vi "Phase III control screen - modified EPV.vi"() -> ()   [LabVIEW 2020]
uses:
  UI Message handler/User Event - Stop/User Event - Stop.lvlib
  UI Message handler/Message Queue/Message Queue.lvlib
  Globals/Phase III Globals.vi
  Controls/boolean ref.ctl
  Controls/Config.ctl
  Controls/EPV .ctl
panel:
  out "Login screen cover":bool
  in  "Log In Tool":bool
  out "User 3":string
  out "User 2":string
  out "State LOX":dbl(knob) caption="Gauge" scale=0.0..40000.0
  out "State ATF":dbl(knob) caption="Gauge" scale=0.0..40000.0
  out "User":string
  in  "C_EPV_124":bool
  out "C_EPV_124 HSS":bool
  in  "C_EPV_16":bool
  in  "N_EPV_202":bool
  in  "C_EPV_1352":bool
  in  "C_EPV_18":bool
  in  "C_EPV_803":bool
  in  "N_EPV_141":bool
  in  "G_EPV_51":bool
  in  "N_EPV_61":bool
  in  "N_EPV_62b":bool
  in  "N_EPV_62a":bool
  in  "C_EPV_127":bool
  in  "C_EPV_123":bool
  in  "C_EPV_8":bool
  in  "C_EPV_7":bool
  in  "C_EPV_2":bool
  in  "F_EPV_75":bool
  in  "N_EPV_206":bool
  in  "N_EPV_203":bool
  in  "F_EPV_28":bool
  in  "F_EPV_142":bool
  in  "F_EPV_ 33":bool
  in  "N_EPV_ 69":bool
  in  "N_EPV_68":bool
  in  "F_EPV_41":bool
  in  "F_EPV_21":bool
  in  "F_EPV_132":bool
  in  "F_EPV_136":bool
  in  "F_EPV_131":bool
  in  "Exit RT":bool
  out "PPSU":bool
  out "RUN ACKNOWLEDGE LOX":bool
  out "Shaft Rotational Direction":string
  out "Speed RPM -lox":dbl format="%#_g r/min"
  out "Frequency":dbl format="%#_g Hz"
  in  "SPEED                      l":dbl format="%#_g r/m"
  in  "RAMP DOWN      l":dbl format="%#_g S"
  in  "RAMP UP             l":dbl format="%#_g S"
  in  "SET FREQ             l":dbl format="%#_g Hz"
  out "RUN ACKNOWLEDGE Atf":bool
  out "Shaft Rotational Direction":string
  out "Speed RPM":dbl format="%#_g r/min"
  out "Frequency":dbl format="%#_g Hz"
  out "Terminal Power":dbl format="%#_g W"
  out "Terminal Current":dbl format="%#_g A"
  out "Terminal Voltage":dbl format="%#_g V"
  out "C_EPV_16 HSS":bool
  out "N_EPV_202 HSS":bool
  out "C_EPV_1352 HSS":bool
  out "C_EPV_18 HSS":bool
  out "C_EPV_803 HSS":bool
  out "N_EPV_141 HSS":bool
  out "G_EPV_51 HSS":bool
  out "N_EPV_61 HSS":bool
  out "N_EPV_62b HSS":bool
  out "N_EPV_62a HSS":bool
  out "C_EPV_127 HSS":bool
  out "C_EPV_123 HSS":bool
  out "C_EPV_8 HSS":bool
  out "C_EPV_7 HSS":bool
  out "C_EPV_2 HSS":bool
  out "N_EPV_75 HSS":bool
  out "N_EPV_206 HSS":bool
  out "N_EPV_203 HSS":bool
  out "F_EPV_28 HSS":bool
  out "N_EPV_142 HSS":bool
  out "F_EPV_33 HSS":bool
  out "N_EPV_69 HSS":bool
  out "N_EPV_68 HSS":bool
  out "F_EPV_41 HSS":bool
  out "F_EPV_21 HSS":bool
  out "F_EPV_132 HSS":bool
  out "F_EPV_136 HSS":bool
  out "F_EPV_131 HSS":bool
  out "MS failure":bool
  out "Over power detection":bool
  out "Over current detection":bool
  out "over voltage detection":bool
  out "power failure status":bool
  out "LOG":bool
  out "TARGET":bool
  out "DR L":bool
  out "DR A":bool
  out "DO":bool
  out "DI":bool
  out "AO":bool
  out "AI":bool
  in  "ADC reset ATF":bool
  in  "MCU reset ATF":bool
  in  "Gate driver ATF":bool
  in  "Motor off ATF":bool
  in  "Motor On ATF":bool
  in  "Update drive ATF":bool
  in  "Adc reset lox":bool
  in  "MCU Reset -LOX":bool
  in  "Gate driver- LOX":bool
  in  "DC off":bool
  in  "DC on":bool
  in  "update ppsu":bool
  in  "Motor Off lox":bool
  in  "Motor On lox":bool
  in  "Update drive lox":bool
  in  "STOP LOG":bool
  in  "SPEED":dbl format="%#_g r/m"
  in  "RAMP DOWN":dbl format="%#_g S"
  in  "RAMP UP":dbl format="%#_g S"
  in  "SET FREQ":dbl format="%#_g Hz"
  in  "SET POWER":dbl format="%#_g W"
  in  "SET CURRENT":dbl format="%#_g A"
  in  "SET VOLTAGE":dbl format="%#_g V"
  in  "OPP(W)":dbl format="%#_g W"
  in  "OCP(A)":dbl format="%#_g A"
  in  "OVP(V)":dbl format="%#_g V"
  in  "Ms initialize":bool
  in  "Alarm ack":bool
  in  "Connect Drive Lox":bool
  in  "Connect Drive ATF":bool
  out "Time Stamp":timestamp format="%<%.3X>T"
  in  "Configure IP":bool
  in  "Datalog phase code":string(combo)
  in  "ABORT":bool
  in  "CONFIGURATION FILE":string(combo)
  in  "IP ADDRESS":string
  in  "HOLD UPDATE":bool
  in  "DAQ SETTING":bool
  in  "Connect ppsu":bool
  in  "Connect RT":bool
  in  "STOP DAQ":bool
  in  "EXIT":bool
  in  "START LOG":bool
  in  "START DAQ":bool
  # "VERSION NUMBER : 1.5"
  # "PHASE III"
  # "RELEASE DATE :10/06/2024"
  # "Select the configuration file"
  # "Select the phase code"
  # "+"
  # "SEQUENCE"
  # "ATF"
  # "LOX"
  # "ENGINE"
  # "EPV CONTROLS"
  # "EPV CONTROLS"
  # "EPV CONTROLS"
  # "Drive ATF Controls"
  # "Drive LOX Controls"
  # "PPSU"
  # "DRIVE ATF"
  # "DRIVE LOX"
  # "PPSU Controls"
  # "PPSU FEEDBACK PARAMETER"
  # "DRIVE ATF SET PARAMETER"
  # "Motor Rotational State"
  # "PPSU SET PARAMETER"
  # "DRIVE LOX SET PARAMETER"
  # "Motor Rotational State"
  # "PPSU FEEDBACK PARAMETER"
  # "DRIVE ATF FEEDBACK PARAMETER"
  # "DRIVE ATF FEEDBACK PARAMETER"
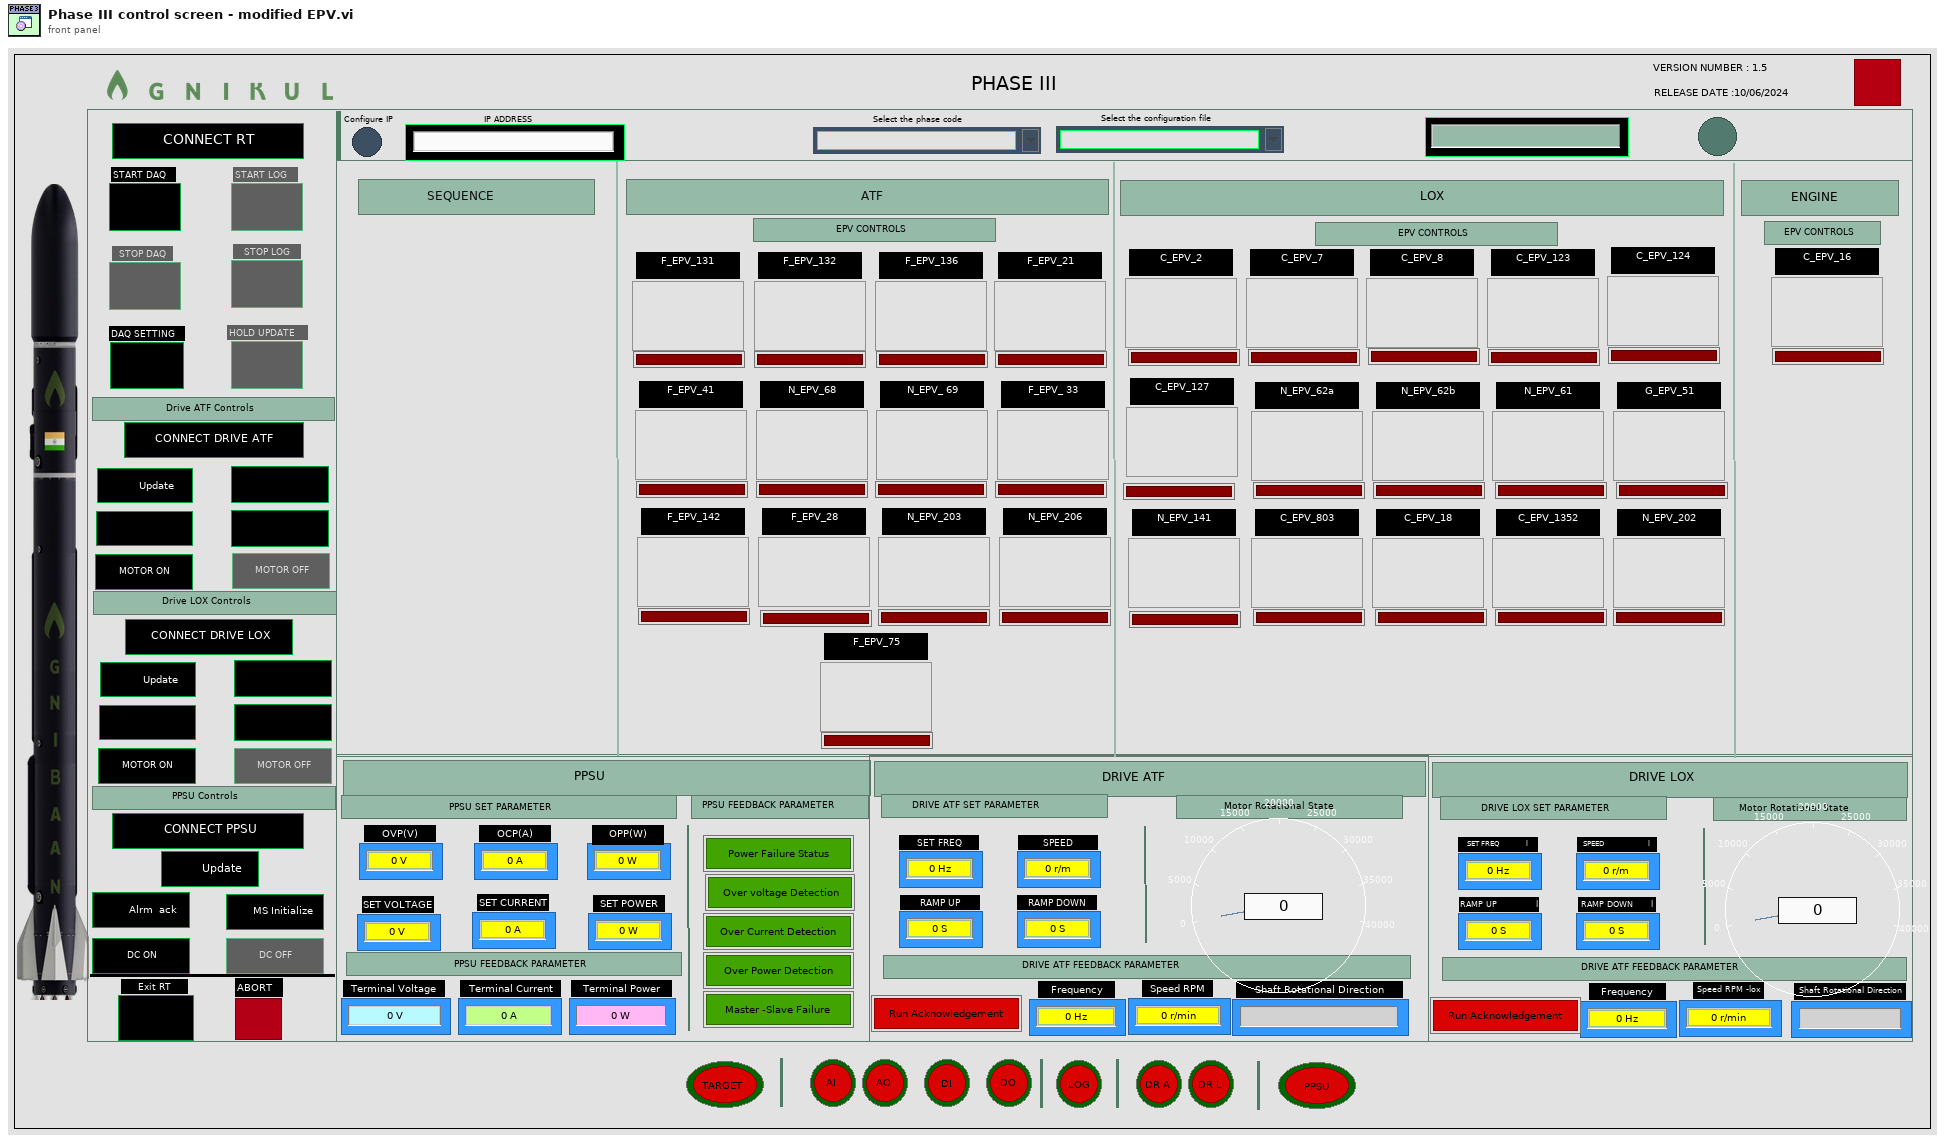
[diagram p1: front panel]
types:
  T1 = typedef "boolean ref.ctl" = cluster{"Connect RT":refnum<vi>, "START DAQ":refnum<vi>, "STOP DAQ":refnum<vi>, "DAQ SETTING":refnum<vi>, "START LOG":refnum<vi>, "STOP LOG":refnum<vi>, "Connect Drive ATF":refnum<vi>, "Update drive ATF":refnum<vi>, "Gate driver ATF":refnum<vi>, "Motor On ATF":refnum<vi>, "ADC reset ATF":refnum<vi>, "Gate driver ATF 2":refnum<vi>, "Motor off ATF":refnum<vi>, "MCU reset ATF":refnum<vi>, "Connect Drive Lox":refnum<vi>, "Update drive lox":refnum<vi>, "Gate driver- LOX":refnum<vi>, "Motor On lox":refnum<vi>, "Adc reset lox":refnum<vi>, "MCU Reset -LOX":refnum<vi>, "Motor Off lox":refnum<vi>, "Connect ppsu":refnum<vi>, "update ppsu":refnum<vi>, "DC on":refnum<vi>, "Alarm ack":refnum<vi>, "DC off":refnum<vi>, "Ms initialize":refnum<vi>, "Exit RT":refnum<vi>, "ABORT":refnum<vi>, "HOLD UPDATE":refnum<vi>}
  T2 = typedef "EPV .ctl" = cluster{"F_EPV_131":refnum<vi>, "F_EPV_132":refnum<vi>, "F_EPV_136":refnum<vi>, "F_EPV_21":refnum<vi>, "F_EPV_41":refnum<vi>, "N_EPV_68":refnum<vi>, "N_EPV_ 69":refnum<vi>, "N_EPV_ 33":refnum<vi>, "F_EPV_142":refnum<vi>, "F_EPV_28":refnum<vi>, "N_EPV_203":refnum<vi>, "N_EPV_206":refnum<vi>, "F_EPV_75":refnum<vi>, "C_EPV_2":refnum<vi>, "C_EPV_7":refnum<vi>, "C_EPV_8":refnum<vi>, "C_EPV_123":refnum<vi>, "C_EPV_124":refnum<vi>, "C_EPV_127":refnum<vi>, "N_EPV_62a":refnum<vi>, "N_EPV_62b":refnum<vi>, "N_EPV_61":refnum<vi>, "G_EPV_51":refnum<vi>, "N_EPV_141":refnum<vi>, "C_EPV_803":refnum<vi>, "C_EPV_18":refnum<vi>, "C_EPV_1352":refnum<vi>, "N_EPV_202":refnum<vi>, "C_EPV_16":refnum<vi>}
  T3 = enum8{"Enabled", "Disabled", "Disabled and Grayed Out"}[]
  T4 = typedef "file folder ctl.ctl" = cluster{"Datalog path":path, "Configuration path":path, "Signal list path":path, "Sub vi's":path, "Authentication":path}
  T5 = typedef "Notifier ctl.ctl" = cluster{"Data":refnum<notifier>}
  T6 = typedef "Message Queue.lvlib/All Message Queues.ctl" = cluster{"UI":refnum<queue>, "NS ":refnum<queue>}
  T7 = typedef "Config.ctl" = cluster{"AO config":cluster{"Channel_Name":string, "Channel_Number":string, "Default_Value":dbl, "Units":string}[], "AI config":cluster{"Channel_Name":string, "Channel_Number":string, "Pre_Scale_min":dbl, "Pre_Scale_max":dbl, "Sensor_min":dbl, "Sensor_max":dbl, "Units":string}[], "DI config":cluster{"Channel_Name":string, "Channel_Number":string, "Default_Value":bool, "DI invert?":bool}[], "DO config":cluster{"Channel_Name":string, "Channel_Number":string, "Default_Value":bool, "DO invert?":bool}[], "TC config":cluster{"Channel_Name":string, "Channel_Number":string, "Pre_Scale_min":dbl, "Pre_Scale_max":dbl, "units":i32, " type":i32}[], "ACC config":cluster{"Channel_Name":string, "Channel_Number":string, "Pre_Scale_min":dbl, "Pre_Scale_max":dbl, "Terminal configuration":i32, "Sensitivity":dbl, "Sensitivity units":i32}[], "SG config":cluster{"Channel_Name":string, "Channel_Number":string, "Pre_Scale_min":dbl, "Pre_Scale_max":dbl}[], "Strain Gauge Settings":cluster{"poisson ratio":dbl, "nominal gage resistance":dbl, "gage factor":dbl}, "Bridge Settings":cluster{"voltage excitation value":dbl, "voltage excitation source":i32, "initial bridge voltage":dbl, "lead wire resistance":dbl, "strain configuration":i32}, "Sample Rate":cluster{"AI Sample Rate":dbl[], "AO Sample Rate":dbl[], "DI Sample Rate":dbl[], "TC Sample Rate":dbl[], "DO Sample Rate":dbl[], "SG Sample Rate":dbl[], "ACC Sample Rate":dbl[]}}
  T8 = enum16{"open", "replace", "create", "open or create", "replace or create", "replace or create with confirmation"}
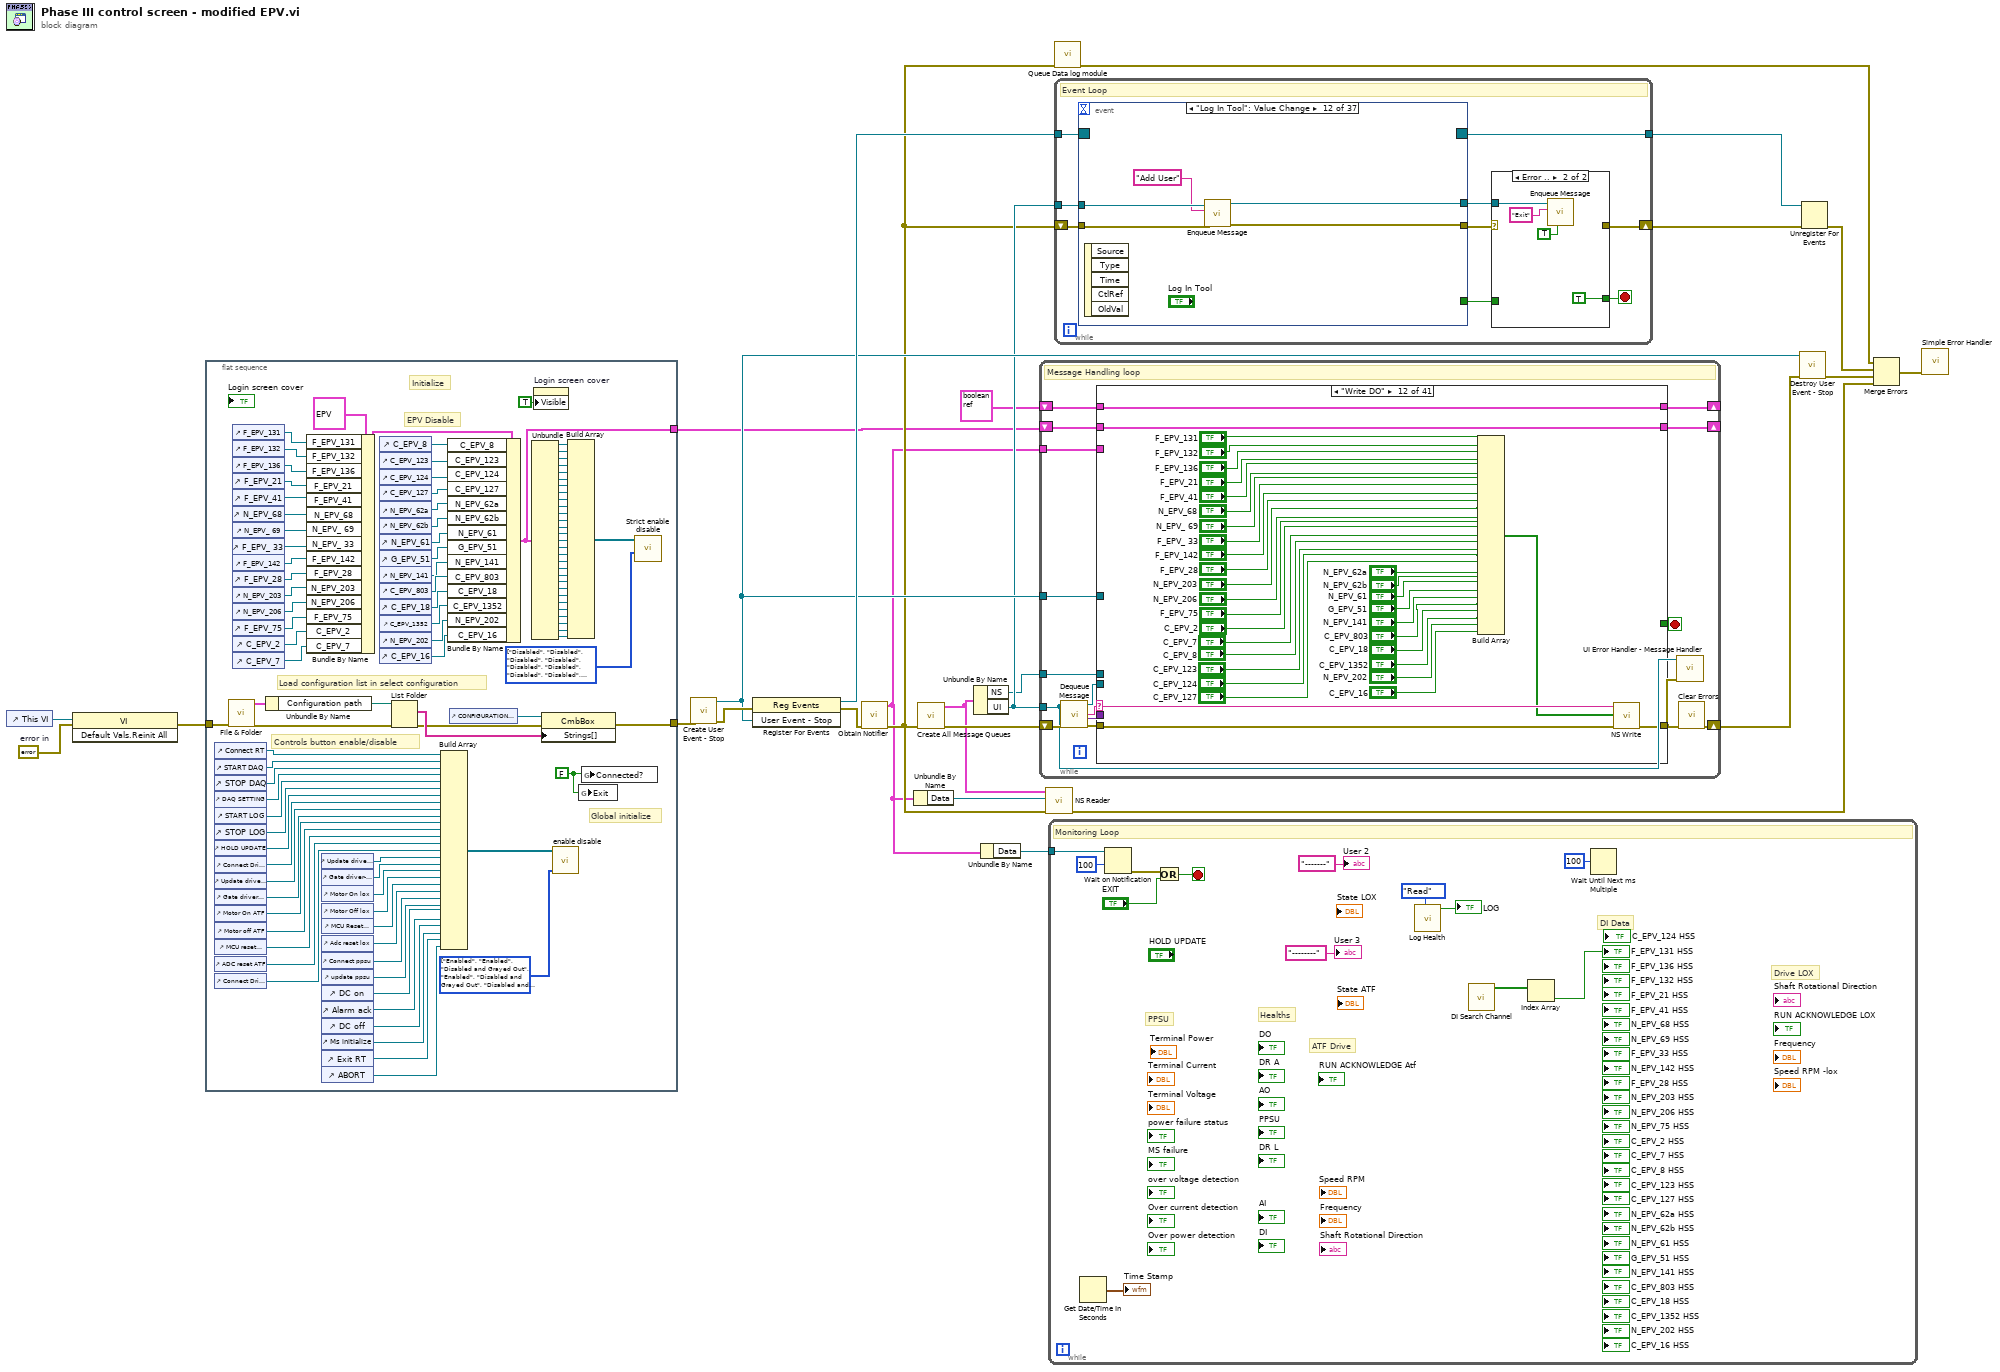
[diagram p0: block diagram]
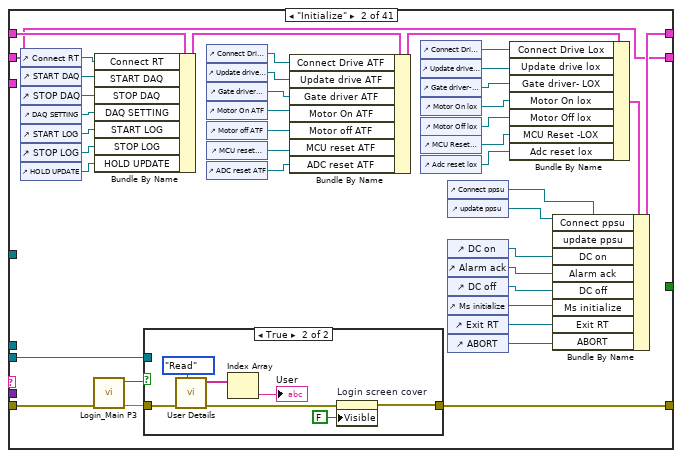
[diagram p3: hidden frame]
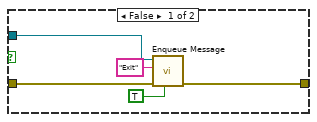
[diagram p4: hidden frame]
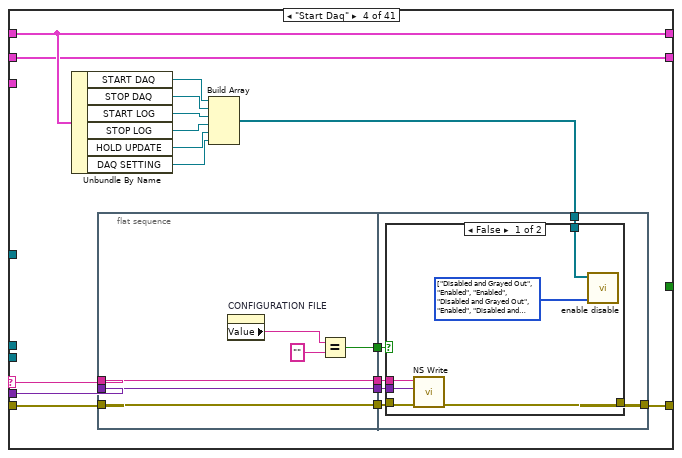
[diagram p6: hidden frame]
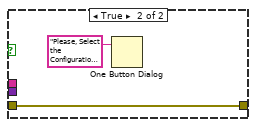
[diagram p7: hidden frame]
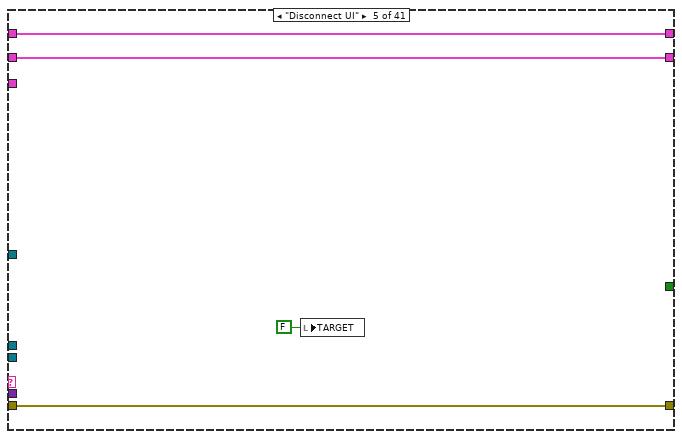
[diagram p8: hidden frame]
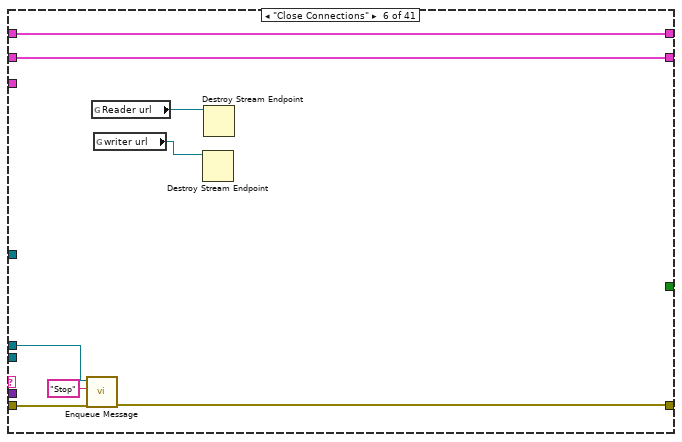
[diagram p9: hidden frame]
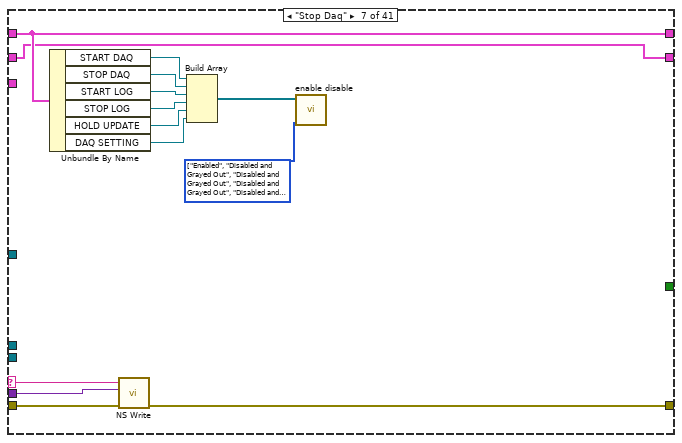
[diagram p10: hidden frame]
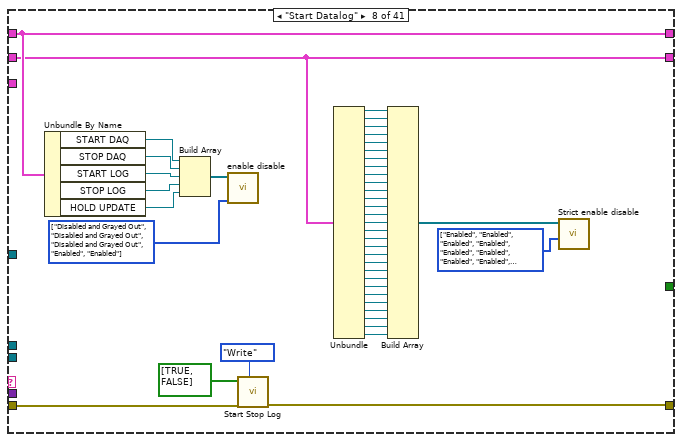
[diagram p11: hidden frame]
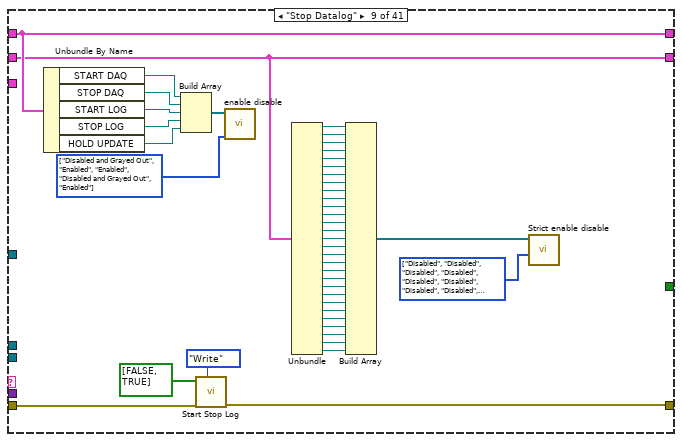
[diagram p12: hidden frame]
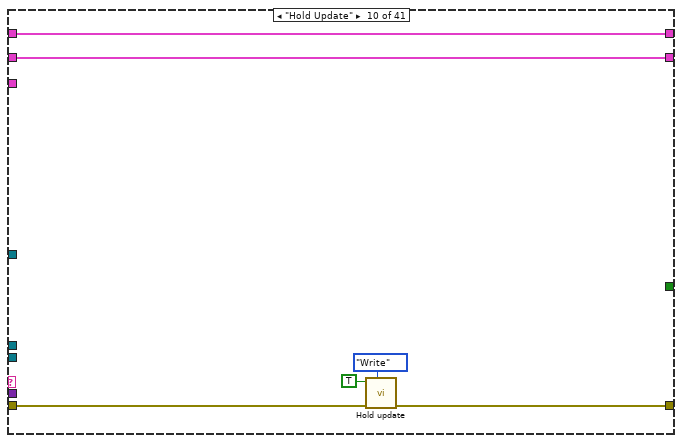
[diagram p13: hidden frame]
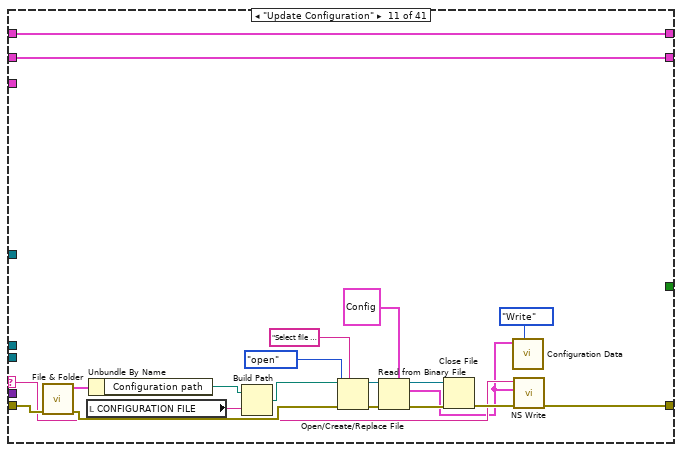
[diagram p14: hidden frame]
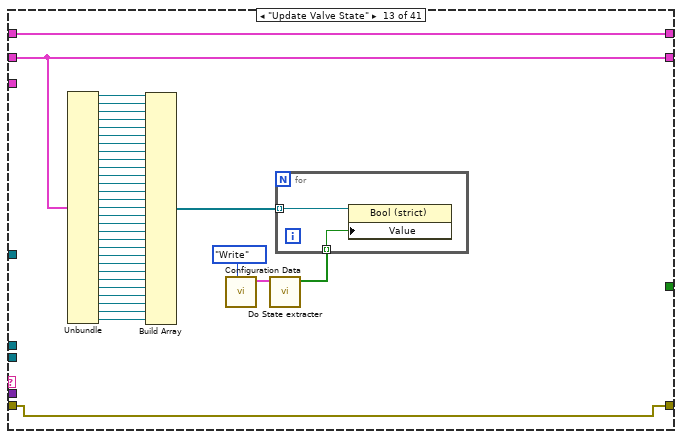
[diagram p15: hidden frame]
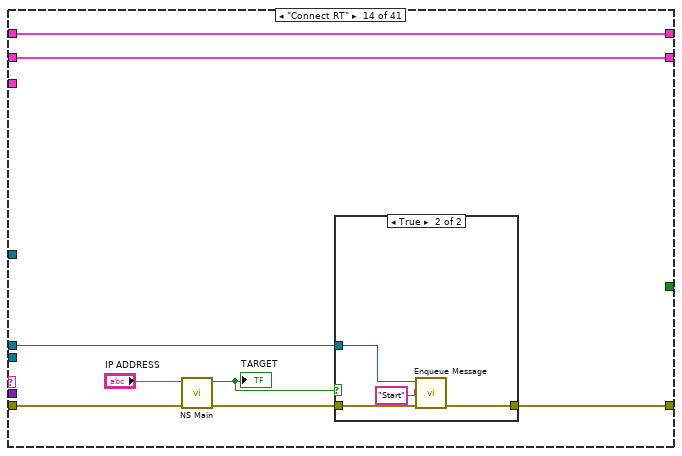
[diagram p16: hidden frame]
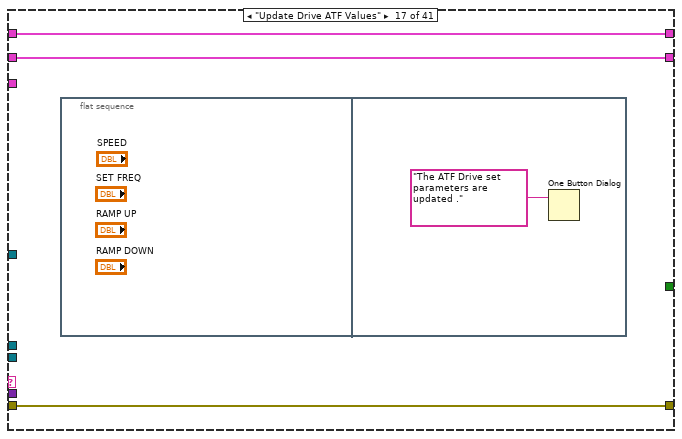
[diagram p20: hidden frame]
diagram:
  w3 = errorcluster {"status"=FALSE, "code"=0, "source"=""}  # error in
  n1 = control-ref of="This VI"() -> (w5:refnum<vi>)
  n2 = invoke class="VI" method="Default Vals.Reinit All"(reference=w5, error in=w3) -> (error out=w2:errorcluster)  [unwired: 1 in, 2 out]
  n3 = flat-sequence {
    tunnel: w2 -> [w127]
    tunnel: [w129] -> w17
    tunnel: [w59] -> w1
    frame #0 {
      w29 = T3 [enum."Enabled", enum."Enabled", enum."Disabled and Grayed Out", enum."Enabled", enum."Disabled and Grayed Out", enum."Disabled and Grayed Out", enum."Disabled and Grayed Out", enum."Enabled", enum."Enabled", enum."Enabled", enum."Enabled", enum."Disabled and Grayed Out", enum."Enabled", enum."Enabled", enum."Enabled", enum."Enabled", enum."Enabled", enum."Enabled", enum."Disabled and Grayed Out", enum."Enabled", enum."Enabled", enum."Enabled", enum."Enabled", enum."Enabled", enum."Enabled", enum."Disabled and Grayed Out", enum."Enabled", enum."Enabled", enum."Enabled"] items=["Enabled", "Disabled", "Disabled and Grayed Out"] ("Disabled")
      w61 = T3 [enum."Disabled", enum."Disabled", enum."Disabled", enum."Disabled", enum."Disabled", enum."Disabled", enum."Disabled", enum."Disabled", enum."Disabled", enum."Disabled", enum."Disabled", enum."Disabled", enum."Disabled", enum."Disabled", enum."Disabled", enum."Disabled", enum."Disabled", enum."Disabled", enum."Disabled", enum."Disabled", enum."Disabled", enum."Disabled", enum."Disabled", enum."Disabled", enum."Disabled", enum."Disabled", enum."Disabled", enum."Disabled", enum."Disabled"] items=["Enabled", "Disabled", "Disabled and Grayed Out"] ("Disabled")
      w130 = FALSE ("Start Data log")
      # "Global initialize"
      # "Load configuration list in select configuration"
      # "Controls button enable/disable"
      # "EPV Disable"
      # "Initialize"
      n4 = control-ref of="Connect RT"() -> (w58:refnum<vi>)
      n5 = control-ref of="START DAQ"() -> (w57:refnum<vi>)
      n6 = control-ref of="STOP DAQ"() -> (w56:refnum<vi>)
      n7 = control-ref of="DAQ SETTING"() -> (w55:refnum<vi>)
      n8 = control-ref of="START LOG"() -> (w54:refnum<vi>)
      n9 = control-ref of="STOP LOG"() -> (w53:refnum<vi>)
      n10 = control-ref of="HOLD UPDATE"() -> (w52:refnum<vi>)
      n11 = control-ref of="Connect Drive ATF"() -> (w51:refnum<vi>)
      n12 = control-ref of="Update drive ATF"() -> (w50:refnum<vi>)
      n13 = control-ref of="Gate driver ATF"() -> (w49:refnum<vi>)
      n14 = control-ref of="Motor On ATF"() -> (w48:refnum<vi>)
      n15 = control-ref of="Motor off ATF"() -> (w47:refnum<vi>)
      n16 = control-ref of="MCU reset ATF"() -> (w46:refnum<vi>)
      n17 = control-ref of="ADC reset ATF"() -> (w45:refnum<vi>)
      n18 = control-ref of="Connect Drive Lox"() -> (w44:refnum<vi>)
      n19 = call "File & Folder.vi"("error in (no error)"=w127) -> ("error out"=w123:errorcluster, "File Output"=w126:T4)  [unwired: 9 in]
      n20 = control-ref of="F_EPV_131"() -> (w63:refnum<vi>)
      n21 = control-ref of="F_EPV_132"() -> (w64:refnum<vi>)
      n22 = control-ref of="F_EPV_136"() -> (w65:refnum<vi>)
      n23 = control-ref of="F_EPV_21"() -> (w66:refnum<vi>)
      n24 = control-ref of="F_EPV_41"() -> (w67:refnum<vi>)
      n25 = control-ref of="N_EPV_68"() -> (w68:refnum<vi>)
      n26 = control-ref of="N_EPV_ 69"() -> (w69:refnum<vi>)
      n27 = control-ref of="F_EPV_ 33"() -> (w70:refnum<vi>)
      n28 = control-ref of="F_EPV_142"() -> (w71:refnum<vi>)
      n29 = control-ref of="F_EPV_28"() -> (w72:refnum<vi>)
      n30 = control-ref of="N_EPV_203"() -> (w73:refnum<vi>)
      n31 = control-ref of="N_EPV_206"() -> (w74:refnum<vi>)
      n32 = control-ref of="F_EPV_75"() -> (w75:refnum<vi>)
      n33 = control-ref of="C_EPV_2"() -> (w76:refnum<vi>)
      n34 = control-ref of="C_EPV_7"() -> (w77:refnum<vi>)
      n35 = Unbundle By Name(w126) -> ("Configuration path"=w125:path)
      n36 = Bundle By Name(cluster=T2 {"F_EPV_131"=refnum, "F_EPV_132"=refnum, "F_EPV_136"=refnum, "F_EPV_21"=refnum, "F_EPV_41"=refnum, "N_EPV_68"=refnum, "N_EPV_ 69"=refnum, "N_EPV_ 33"=refnum, "F_EPV_142"=refnum, "F_EPV_28"=refnum, "N_EPV_203"=refnum, "N_EPV_206"=refnum, "F_EPV_75"=refnum, "C_EPV_2"=refnum, "C_EPV_7"=refnum, "C_EPV_8"=refnum, "C_EPV_123"=refnum, "C_EPV_124"=refnum, "C_EPV_127"=refnum, "N_EPV_62a"=refnum, "N_EPV_62b"=refnum, "N_EPV_61"=refnum, "G_EPV_51"=refnum, "N_EPV_141"=refnum, "C_EPV_803"=refnum, "C_EPV_18"=refnum, "C_EPV_1352"=refnum, "N_EPV_202"=refnum, "C_EPV_16"=refnum} ("Cluster"), "F_EPV_131"=w63, "F_EPV_132"=w64, "F_EPV_136"=w65, "F_EPV_21"=w66, "F_EPV_41"=w67, "N_EPV_68"=w68, "N_EPV_ 69"=w69, "N_EPV_ 33"=w70, "F_EPV_142"=w71, "F_EPV_28"=w72, "N_EPV_203"=w73, "N_EPV_206"=w74, "F_EPV_75"=w75, "C_EPV_2"=w76, "C_EPV_7"=w77) -> (w78:T2)
      n37 = control-ref of="Update drive lox"() -> (w43:refnum<vi>)
      n38 = control-ref of="Gate driver- LOX"() -> (w42:refnum<vi>)
      n39 = control-ref of="Motor On lox"() -> (w41:refnum<vi>)
      n40 = control-ref of="Motor Off lox"() -> (w40:refnum<vi>)
      n41 = control-ref of="MCU Reset -LOX"() -> (w39:refnum<vi>)
      n42 = control-ref of="Adc reset lox"() -> (w38:refnum<vi>)
      n43 = control-ref of="Connect ppsu"() -> (w37:refnum<vi>)
      n44 = control-ref of="update ppsu"() -> (w36:refnum<vi>)
      n45 = control-ref of="DC on"() -> (w35:refnum<vi>)
      n46 = control-ref of="Alarm ack"() -> (w34:refnum<vi>)
      n47 = control-ref of="DC off"() -> (w33:refnum<vi>)
      n48 = control-ref of="Ms initialize"() -> (w32:refnum<vi>)
      n49 = control-ref of="Exit RT"() -> (w31:refnum<vi>)
      n50 = control-ref of="ABORT"() -> (w30:refnum<vi>)
      n51 = control-ref of="C_EPV_8"() -> (w79:refnum<vi>)
      n52 = control-ref of="C_EPV_123"() -> (w80:refnum<vi>)
      n53 = control-ref of="C_EPV_124"() -> (w81:refnum<vi>)
      n54 = control-ref of="C_EPV_127"() -> (w82:refnum<vi>)
      n55 = control-ref of="N_EPV_62a"() -> (w83:refnum<vi>)
      n56 = control-ref of="N_EPV_62b"() -> (w84:refnum<vi>)
      n57 = control-ref of="N_EPV_61"() -> (w85:refnum<vi>)
      n58 = control-ref of="G_EPV_51"() -> (w86:refnum<vi>)
      n59 = control-ref of="N_EPV_141"() -> (w87:refnum<vi>)
      n60 = control-ref of="C_EPV_803"() -> (w88:refnum<vi>)
      n61 = control-ref of="C_EPV_18"() -> (w89:refnum<vi>)
      n62 = control-ref of="C_EPV_1352"() -> (w90:refnum<vi>)
      n63 = control-ref of="N_EPV_202"() -> (w91:refnum<vi>)
      n64 = control-ref of="C_EPV_16"() -> (w92:refnum<vi>)
      n65 = List Folder(path=w125, error in=w123) -> (filenames=w124:string[], error out=w122:errorcluster)  [unwired: 2 in, 2 out]
      n66 = Build Array(w58, w57, w56, w55, w54, w53, w52, w51, w50, w49, w48, w47, w46, w45, w44, w43, w42, w41, w40, w39, w38, w37, w36, w35, w34, w33, w32, w31, w30) -> (w28:refnum<vi>[])
      n67 = Bundle By Name(cluster=w78, "C_EPV_8"=w79, "C_EPV_123"=w80, "C_EPV_124"=w81, "C_EPV_127"=w82, "N_EPV_62a"=w83, "N_EPV_62b"=w84, "N_EPV_61"=w85, "G_EPV_51"=w86, "N_EPV_141"=w87, "C_EPV_803"=w88, "C_EPV_18"=w89, "C_EPV_1352"=w90, "N_EPV_202"=w91, "C_EPV_16"=w92) -> (w59:T2)
      n68 = control-ref of="CONFIGURATION FILE"() -> (w128:refnum<vi>)
      n69 = Unbundle(w59) -> ("F_EPV_131"=w93:refnum<vi>, "F_EPV_132"=w94:refnum<vi>, "F_EPV_136"=w95:refnum<vi>, "F_EPV_21"=w96:refnum<vi>, "F_EPV_41"=w97:refnum<vi>, "N_EPV_68"=w98:refnum<vi>, "N_EPV_ 69"=w99:refnum<vi>, "N_EPV_ 33"=w100:refnum<vi>, "F_EPV_142"=w101:refnum<vi>, "F_EPV_28"=w102:refnum<vi>, "N_EPV_203"=w103:refnum<vi>, "N_EPV_206"=w104:refnum<vi>, "F_EPV_75"=w105:refnum<vi>, "C_EPV_2"=w106:refnum<vi>, "C_EPV_7"=w107:refnum<vi>, "C_EPV_8"=w108:refnum<vi>, "C_EPV_123"=w109:refnum<vi>, "C_EPV_124"=w110:refnum<vi>, "C_EPV_127"=w111:refnum<vi>, "N_EPV_62a"=w112:refnum<vi>, "N_EPV_62b"=w113:refnum<vi>, "N_EPV_61"=w114:refnum<vi>, "G_EPV_51"=w115:refnum<vi>, "N_EPV_141"=w116:refnum<vi>, "C_EPV_803"=w117:refnum<vi>, "C_EPV_18"=w118:refnum<vi>, "C_EPV_1352"=w119:refnum<vi>, "N_EPV_202"=w120:refnum<vi>, "C_EPV_16"=w121:refnum<vi>)
      n70 = property on="Login screen cover" class="Bool (strict)"("Visible"=TRUE) -> ()  [unwired: 2 in, 2 out]
      n71 = property class="CmbBox"(reference=w128, error in=w122, "Strings[]"=w124) -> (error out=w129:errorcluster)  [unwired: 1 out]
      n72 = call "enable disable.vi"("Disabled"=w29, "ref in"=w28) -> ()  [unwired: 10 in]
      n73 = Build Array(w93, w94, w95, w96, w97, w98, w99, w100, w101, w102, w103, w104, w105, w106, w107, w108, w109, w110, w111, w112, w113, w114, w115, w116, w117, w118, w119, w120, w121) -> (w60:refnum<vi>[])
      n74 = global write "Phase III Globals.vi" "Exit"(w130) -> ()
      n75 = global write "Phase III Globals.vi" "Connected?"(w130) -> ()
      n76 = call "Strict enable disable.vi"("Disabled"=w61, "Ref in"=w60) -> ()  [unwired: 10 in]
    }
  }
  n77 = call "Create User Event - Stop.vi"("error in (no error)"=w17) -> ("error out"=w23:errorcluster, "User Event - Stop"=w21:refnum<user-event>)  [unwired: 9 in]
  n78 = register-events(error in=w23, w21) -> (reference out=w26:refnum<event-registration>, error out=w16:errorcluster)  [unwired: 1 in]
  n79 = call "Obtain Notifier.vi"("error in"=w16) -> ("error out"=w9:errorcluster, "Notifier Out"=w6:T5)  [unwired: 9 in]
  n80 = Unbundle By Name(w6) -> ("Data"=w10:refnum<notifier>)
  n81 = call "Create All Message Queues.vi"("error in (no error)"=w9) -> ("error out"=w20:errorcluster, "Message Queues out"=w11:T6)  [unwired: 9 in]
  n82 = Unbundle By Name(w11) -> ("NS"=w7:refnum<queue>, "UI"=w19:refnum<queue>)
  n83 = Unbundle By Name(w6) -> ("Data"=w15:refnum<notifier>)
  n84 = while {
    shift-right: [w146] -> w14
    shift-left: w20 -> [w143]
    tunnel: w21 -> [w144]
    tunnel: w19 -> [w136]
    tunnel: w7 -> [w138]
    tunnel: w6 -> [w137]
    shift-right: [w133] -> _
    shift-left: T1 {"Connect RT"=refnum, "START DAQ"=refnum, "STOP DAQ"=refnum, "DAQ SETTING"=refnum, "START LOG"=refnum, "STOP LOG"=refnum, "Connect Drive ATF"=refnum, "Update drive ATF"=refnum, "Gate driver ATF"=refnum, "Motor On ATF"=refnum, "ADC reset ATF"=refnum, "Gate driver ATF 2"=refnum, "Motor off ATF"=refnum, "MCU reset ATF"=refnum, "Connect Drive Lox"=refnum, "Update drive lox"=refnum, "Gate driver- LOX"=refnum, "Motor On lox"=refnum, "Adc reset lox"=refnum, "MCU Reset -LOX"=refnum, "Motor Off lox"=refnum, "Connect ppsu"=refnum, "update ppsu"=refnum, "DC on"=refnum, "Alarm ack"=refnum, "DC off"=refnum, "Ms initialize"=refnum, "Exit RT"=refnum, "ABORT"=refnum, "HOLD UPDATE"=refnum} ("Cluster") -> [w134]
    shift-right: [w131] -> _
    shift-left: w1 -> [w132]
    stop <- w145 stop-if-true
    # "Message Handling loop"
    n85 = call "Dequeue Message.vi"("error in (no error)"=w143, "Message Queue"=w136) -> ("error out"=w142:errorcluster, "Message Data"=w139:variant, "Message"=w141:string, "dup Message Queue"=w140:refnum<queue>)  [unwired: 6 in]
    n86 = case shown="\"Write DO\"" w141 {
      selector: w141 -> [_ _ _ w220 _ _ w265 _ _ _ w365 w414 _ _ _ _ _ _ _ _ _ _ _ _ _ _ _ _ _ _ _ _ _ _ _ _ _ _ _ _ _]
      tunnel: w142 -> [w149 w154 w204 w219 w245 w249 w264 w271 w315 w360 w376 w416 w452 w462 w470 w473 w476 w480 w484 w487 w490 w501 w512 w515 w518 w521 w532 w543 w546 w556 w566 w569 w573 w576 w579 w585 w599 w605 w624 w627 w629]
      tunnel: [w149 w151 w204 w218 w245 w247 w267 w270 w314 w359 w366 w415 w452 w457 w470 w473 w476 w480 w484 w487 w490 w501 w512 w515 w518 w521 w532 w543 w546 w556 w566 w569 w573 w576 w579 w592 w598 w603 w613 w627 w628] -> w135
      tunnel: [_ _ _ _ _ _ _ _ _ _ _ _ _ _ _ _ _ _ _ _ _ _ _ _ _ _ _ _ _ _ _ _ _ _ _ TRUE ("EXIT") _ _ _ _ _] -> w145
      tunnel: w144 -> [_ _ _ _ _ _ _ _ _ _ _ _ _ _ _ _ _ _ _ _ _ _ _ _ _ _ _ _ _ _ _ _ _ _ _ w594 _ _ _ _ _]
      tunnel: w140 -> [_ w150 _ _ _ _ _ _ _ _ _ _ _ _ _ _ _ _ _ _ _ _ _ _ _ _ _ _ _ _ _ _ _ _ _ w593 _ _ _ _ _]
      tunnel: w139 -> [_ _ _ w221 _ _ w266 _ _ _ _ _ _ _ _ _ _ _ _ _ _ _ _ _ _ _ _ _ _ _ _ _ _ _ _ _ _ _ _ _ _]
      tunnel: w138 -> [_ _ _ _ _ w248 _ _ _ _ _ _ _ w459 _ _ _ _ _ _ _ _ _ _ _ _ _ _ _ _ _ _ _ _ _ w583 _ _ _ _ _]
      tunnel: w137 -> [_ _ _ _ _ _ _ _ _ _ _ _ _ _ _ _ _ _ _ _ _ _ _ _ _ _ _ _ _ _ _ _ _ _ _ w590 _ _ _ _ _]
      tunnel: w134 -> [w148 w189 w203 w217 w243 w251 w256 w304 w349 w361 w381 w412 w451 w456 w469 w472 w475 w479 w483 w486 w489 w500 w504 w514 w517 w520 w531 w534 w545 w555 w558 w568 w572 w575 w578 w581 w601 w607 w618 w626 w631]
      tunnel: [w148 w164 w203 w217 w243 w251 w256 w304 w349 w361 w381 w412 w451 w456 w469 w472 w475 w479 w483 w486 w489 w500 w504 w514 w517 w520 w531 w534 w545 w555 w558 w568 w572 w575 w578 w581 w601 w607 w618 w626 w631] -> w133
      tunnel: w132 -> [w147 w155 w202 w205 w242 w246 w254 w303 w347 w356 w362 w382 w417 w455 w468 w471 w474 w478 w482 w485 w488 w491 w502 w513 w516 w519 w522 w533 w544 w547 w557 w567 w571 w574 w577 w580 w596 w602 w612 w625 w630]
      tunnel: [w147 w155 w202 w205 w242 w246 w254 w303 w347 w356 w362 w382 w417 w455 w468 w471 w474 w478 w482 w485 w488 w491 w502 w513 w516 w519 w522 w533 w544 w547 w557 w567 w571 w574 w577 w580 w596 w602 w612 w625 w630] -> w131
      frame "Pole event", Default {
      }
      frame "Initialize" {
        n87 = control-ref of="Connect RT"() -> (w187:refnum<vi>)
        n88 = control-ref of="START DAQ"() -> (w186:refnum<vi>)
        n89 = control-ref of="STOP DAQ"() -> (w185:refnum<vi>)
        n90 = control-ref of="DAQ SETTING"() -> (w184:refnum<vi>)
        n91 = control-ref of="START LOG"() -> (w183:refnum<vi>)
        n92 = control-ref of="STOP LOG"() -> (w182:refnum<vi>)
        n93 = control-ref of="HOLD UPDATE"() -> (w181:refnum<vi>)
        n94 = call "Login_Main P3.vi"(8:w154) -> (0:w152, "Login pass"=w153:bool)  [unwired: 9 in]
        n95 = Bundle By Name(cluster=w189, "Connect RT"=w187, "START DAQ"=w186, "STOP DAQ"=w185, "DAQ SETTING"=w184, "START LOG"=w183, "STOP LOG"=w182, "HOLD UPDATE"=w181) -> (w188:T1)
        n96 = case shown="True" w153 {
          tunnel: w152 -> [w194 w201]
          tunnel: [w193 w195] -> w151
          tunnel: w150 -> [w192 _]
          frame False {
            n97 = call "Enqueue Message.vi"("Priority Message? (F)"=TRUE, "error in (no error)"=w194, "Message"="Exit", "Message Queue"=w192) -> ("error out"=w193:errorcluster)  [unwired: 6 in, 1 out]
          }
          frame True {
            n98 = call "User Details.vi"("Enum"=enum16{"Read", "Write"}."Read", "error in"=w201) -> ("error out"=w197:errorcluster, "User details R"=w199:string[])  [unwired: 8 in]
            n99 = Index Array(array=w199) -> (element=→"User":string)  [unwired: 1 in]
            n100 = property on="Login screen cover" class="Bool (strict)"(error in=w197, "Visible"=FALSE) -> (error out=w195:errorcluster)  [unwired: 1 in, 1 out]
          }
        }
        n101 = control-ref of="Connect Drive ATF"() -> (w179:refnum<vi>)
        n102 = control-ref of="Update drive ATF"() -> (w178:refnum<vi>)
        n103 = control-ref of="Gate driver ATF"() -> (w177:refnum<vi>)
        n104 = control-ref of="Motor On ATF"() -> (w176:refnum<vi>)
        n105 = control-ref of="Motor off ATF"() -> (w175:refnum<vi>)
        n106 = control-ref of="MCU reset ATF"() -> (w174:refnum<vi>)
        n107 = control-ref of="ADC reset ATF"() -> (w173:refnum<vi>)
        n108 = Bundle By Name(cluster=w188, "Connect Drive ATF"=w179, "Update drive ATF"=w178, "Gate driver ATF"=w177, "Motor On ATF"=w176, "Motor off ATF"=w175, "MCU reset ATF"=w174, "ADC reset ATF"=w173) -> (w180:T1)
        n109 = control-ref of="Connect Drive Lox"() -> (w172:refnum<vi>)
        n110 = control-ref of="Update drive lox"() -> (w171:refnum<vi>)
        n111 = control-ref of="Gate driver- LOX"() -> (w170:refnum<vi>)
        n112 = control-ref of="Motor On lox"() -> (w169:refnum<vi>)
        n113 = control-ref of="Motor Off lox"() -> (w168:refnum<vi>)
        n114 = control-ref of="MCU Reset -LOX"() -> (w167:refnum<vi>)
        n115 = control-ref of="Adc reset lox"() -> (w166:refnum<vi>)
        n116 = control-ref of="Connect ppsu"() -> (w163:refnum<vi>)
        n117 = control-ref of="update ppsu"() -> (w162:refnum<vi>)
        n118 = control-ref of="DC on"() -> (w161:refnum<vi>)
        n119 = control-ref of="Alarm ack"() -> (w160:refnum<vi>)
        n120 = control-ref of="DC off"() -> (w159:refnum<vi>)
        n121 = control-ref of="Ms initialize"() -> (w158:refnum<vi>)
        n122 = control-ref of="Exit RT"() -> (w157:refnum<vi>)
        n123 = control-ref of="ABORT"() -> (w156:refnum<vi>)
        n124 = Bundle By Name(cluster=w180, "Connect Drive Lox"=w172, "Update drive lox"=w171, "Gate driver- LOX"=w170, "Motor On lox"=w169, "Motor Off lox"=w168, "MCU Reset -LOX"=w167, "Adc reset lox"=w166) -> (w165:T1)
        n125 = Bundle By Name(cluster=w165, "Connect ppsu"=w163, "update ppsu"=w162, "DC on"=w161, "Alarm ack"=w160, "DC off"=w159, "Ms initialize"=w158, "Exit RT"=w157, "ABORT"=w156) -> (w164:T1)
      }
      frame "Ip Config" {
      }
      frame "Start Daq" {
        n126 = Unbundle By Name(w217) -> ("START DAQ"=w216:refnum<vi>, "STOP DAQ"=w215:refnum<vi>, "START LOG"=w214:refnum<vi>, "STOP LOG"=w213:refnum<vi>, "HOLD UPDATE"=w212:refnum<vi>, "DAQ SETTING"=w211:refnum<vi>)
        n127 = flat-sequence {
          tunnel: w219 -> [w225]
          tunnel: w220 -> [w226]
          tunnel: w221 -> [w227]
          tunnel: [w227] -> w210
          tunnel: [w226] -> w209
          tunnel: [w225] -> w208
          tunnel: [w222] -> w207
          tunnel: [w230] -> w218
          tunnel: w210 -> [w233]
          tunnel: w209 -> [w232]
          tunnel: w208 -> [w231]
          tunnel: w207 -> [w229]
          tunnel: w206 -> [w228]
          frame #0 {
            n128 = property on="CONFIGURATION FILE" class="CmbBox"() -> ("Value"=w224:string)  [unwired: 2 in, 2 out]
            n129 = Equal?(x=w224, y="") -> (x = y?=w222:bool)
          }
          frame #1 {
            n130 = case shown="False" w229 {
              tunnel: w233 -> [w239 _]
              tunnel: w232 -> [w238 _]
              tunnel: w231 -> [w237 w241]
              tunnel: [w236 w241] -> w230
              tunnel: w228 -> [w235 _]
              frame False {
                w234 = T3 [enum."Disabled and Grayed Out", enum."Enabled", enum."Enabled", enum."Disabled and Grayed Out", enum."Enabled", enum."Disabled and Grayed Out"] items=["Enabled", "Disabled", "Disabled and Grayed Out"] ("Disabled")
                n131 = call "NS Write.vi"("error in"=w237, "Data"=w239, "Message"=w238) -> ("error out"=w236:errorcluster)  [unwired: 8 in]
                n132 = call "enable disable.vi"("Disabled"=w234, "ref in"=w235) -> ()  [unwired: 10 in]
              }
              frame True {
                n133 = One Button Dialog(message="Please, Select the Configuration File !!") -> ()  [unwired: 1 in, 1 out]
              }
            }
          }
        }
        n134 = Build Array(w216, w215, w214, w213, w212, w211) -> (w206:refnum<vi>[])
      }
      frame "Disconnect UI" {
        n135 = local write "TARGET"(FALSE ("TARGET")) -> ()
      }
      frame "Close Connections" {
        n136 = call "Enqueue Message.vi"("error in (no error)"=w249, "Message"="Stop", "Message Queue"=w248) -> ("error out"=w247:errorcluster)  [unwired: 7 in, 1 out]
        n137 = global read "Phase III Globals.vi" "Reader url"() -> (w253:refnum<k21>)
        n138 = global read "Phase III Globals.vi" "writer url"() -> (w252:refnum<k21>)
        n139 = Destroy Stream Endpoint(11:w252) -> ()  [unwired: 1 in, 1 out]
        n140 = Destroy Stream Endpoint(11:w253) -> ()  [unwired: 1 in, 1 out]
      }
      frame "Stop Daq" {
        w257 = T3 [enum."Enabled", enum."Disabled and Grayed Out", enum."Disabled and Grayed Out", enum."Disabled and Grayed Out", enum."Disabled and Grayed Out", enum."Enabled"] items=["Enabled", "Disabled", "Disabled and Grayed Out"] ("Disabled")
        n141 = Unbundle By Name(w256) -> ("START DAQ"=w263:refnum<vi>, "STOP DAQ"=w262:refnum<vi>, "START LOG"=w261:refnum<vi>, "STOP LOG"=w260:refnum<vi>, "HOLD UPDATE"=w258:refnum<vi>, "DAQ SETTING"=w255:refnum<vi>)
        n142 = call "NS Write.vi"("error in"=w264, "Data"=w266, "Message"=w265) -> ("error out"=w267:errorcluster)  [unwired: 8 in]
        n143 = Build Array(w263, w262, w261, w260, w258, w255) -> (w259:refnum<vi>[])
        n144 = call "enable disable.vi"("Disabled"=w257, "ref in"=w259) -> ()  [unwired: 10 in]
      }
      frame "Start Datalog" {
        w273 = T3 [enum."Enabled", enum."Enabled", enum."Enabled", enum."Enabled", enum."Enabled", enum."Enabled", enum."Enabled", enum."Enabled", enum."Enabled", enum."Enabled", enum."Enabled", enum."Enabled", enum."Enabled", enum."Enabled", enum."Enabled", enum."Enabled", enum."Enabled", enum."Enabled", enum."Enabled", enum."Enabled", enum."Enabled", enum."Enabled", enum."Enabled", enum."Enabled", enum."Enabled", enum."Enabled", enum."Enabled", enum."Enabled", enum."Enabled"] items=["Enabled", "Disabled", "Disabled and Grayed Out"] ("Disabled")
        w305 = T3 [enum."Disabled and Grayed Out", enum."Disabled and Grayed Out", enum."Disabled and Grayed Out", enum."Enabled", enum."Enabled"] items=["Enabled", "Disabled", "Disabled and Grayed Out"] ("Disabled")
        n145 = Unbundle By Name(w304) -> ("START DAQ"=w311:refnum<vi>, "STOP DAQ"=w310:refnum<vi>, "START LOG"=w309:refnum<vi>, "STOP LOG"=w308:refnum<vi>, "HOLD UPDATE"=w306:refnum<vi>)
        n146 = Build Array(w311, w310, w309, w308, w306) -> (w307:refnum<vi>[])
        n147 = call "enable disable.vi"("Disabled"=w305, "ref in"=w307) -> ()  [unwired: 10 in]
        n148 = call "Start Stop Log.vi"("Enum"=enum16{"Read", "Write"}."Write", "error in"=w271, "Start Stop log"=bool[] [TRUE, FALSE]) -> ("error out"=w270:errorcluster)  [unwired: 7 in, 1 out]
        n149 = Unbundle(w303) -> ("F_EPV_131"=w302:refnum<vi>, "F_EPV_132"=w301:refnum<vi>, "F_EPV_136"=w300:refnum<vi>, "F_EPV_21"=w299:refnum<vi>, "F_EPV_41"=w298:refnum<vi>, "N_EPV_68"=w297:refnum<vi>, "N_EPV_ 69"=w296:refnum<vi>, "N_EPV_ 33"=w295:refnum<vi>, "F_EPV_142"=w294:refnum<vi>, "F_EPV_28"=w293:refnum<vi>, "N_EPV_203"=w292:refnum<vi>, "N_EPV_206"=w291:refnum<vi>, "F_EPV_75"=w290:refnum<vi>, "C_EPV_2"=w289:refnum<vi>, "C_EPV_7"=w288:refnum<vi>, "C_EPV_8"=w287:refnum<vi>, "C_EPV_123"=w286:refnum<vi>, "C_EPV_124"=w285:refnum<vi>, "C_EPV_127"=w284:refnum<vi>, "N_EPV_62a"=w283:refnum<vi>, "N_EPV_62b"=w282:refnum<vi>, "N_EPV_61"=w281:refnum<vi>, "G_EPV_51"=w280:refnum<vi>, "N_EPV_141"=w279:refnum<vi>, "C_EPV_803"=w278:refnum<vi>, "C_EPV_18"=w277:refnum<vi>, "C_EPV_1352"=w276:refnum<vi>, "N_EPV_202"=w275:refnum<vi>, "C_EPV_16"=w274:refnum<vi>)
        n150 = Build Array(w302, w301, w300, w299, w298, w297, w296, w295, w294, w293, w292, w291, w290, w289, w288, w287, w286, w285, w284, w283, w282, w281, w280, w279, w278, w277, w276, w275, w274) -> (w272:refnum<vi>[])
        n151 = call "Strict enable disable.vi"("Disabled"=w273, "Ref in"=w272) -> ()  [unwired: 10 in]
      }
      frame "Stop Datalog" {
        w316 = T3 [enum."Disabled", enum."Disabled", enum."Disabled", enum."Disabled", enum."Disabled", enum."Disabled", enum."Disabled", enum."Disabled", enum."Disabled", enum."Disabled", enum."Disabled", enum."Disabled", enum."Disabled", enum."Disabled", enum."Disabled", enum."Disabled", enum."Disabled", enum."Disabled", enum."Disabled", enum."Disabled", enum."Disabled", enum."Disabled", enum."Disabled", enum."Disabled", enum."Disabled", enum."Disabled", enum."Disabled", enum."Disabled", enum."Disabled"] items=["Enabled", "Disabled", "Disabled and Grayed Out"] ("Disabled")
        w350 = T3 [enum."Disabled and Grayed Out", enum."Enabled", enum."Enabled", enum."Disabled and Grayed Out", enum."Enabled"] items=["Enabled", "Disabled", "Disabled and Grayed Out"] ("Disabled")
        n152 = Unbundle By Name(w349) -> ("START DAQ"=w348:refnum<vi>, "STOP DAQ"=w355:refnum<vi>, "START LOG"=w354:refnum<vi>, "STOP LOG"=w353:refnum<vi>, "HOLD UPDATE"=w351:refnum<vi>)
        n153 = Build Array(w348, w355, w354, w353, w351) -> (w352:refnum<vi>[])
        n154 = call "Start Stop Log.vi"("Enum"=enum16{"Read", "Write"}."Write", "error in"=w315, "Start Stop log"=bool[] [FALSE, TRUE]) -> ("error out"=w314:errorcluster)  [unwired: 7 in, 1 out]
        n155 = call "enable disable.vi"("Disabled"=w350, "ref in"=w352) -> ()  [unwired: 10 in]
        n156 = Unbundle(w347) -> ("F_EPV_131"=w346:refnum<vi>, "F_EPV_132"=w345:refnum<vi>, "F_EPV_136"=w344:refnum<vi>, "F_EPV_21"=w343:refnum<vi>, "F_EPV_41"=w342:refnum<vi>, "N_EPV_68"=w341:refnum<vi>, "N_EPV_ 69"=w340:refnum<vi>, "N_EPV_ 33"=w339:refnum<vi>, "F_EPV_142"=w338:refnum<vi>, "F_EPV_28"=w337:refnum<vi>, "N_EPV_203"=w336:refnum<vi>, "N_EPV_206"=w335:refnum<vi>, "F_EPV_75"=w334:refnum<vi>, "C_EPV_2"=w333:refnum<vi>, "C_EPV_7"=w332:refnum<vi>, "C_EPV_8"=w331:refnum<vi>, "C_EPV_123"=w330:refnum<vi>, "C_EPV_124"=w329:refnum<vi>, "C_EPV_127"=w328:refnum<vi>, "N_EPV_62a"=w327:refnum<vi>, "N_EPV_62b"=w326:refnum<vi>, "N_EPV_61"=w325:refnum<vi>, "G_EPV_51"=w324:refnum<vi>, "N_EPV_141"=w323:refnum<vi>, "C_EPV_803"=w322:refnum<vi>, "C_EPV_18"=w321:refnum<vi>, "C_EPV_1352"=w320:refnum<vi>, "N_EPV_202"=w319:refnum<vi>, "C_EPV_16"=w318:refnum<vi>)
        n157 = Build Array(w346, w345, w344, w343, w342, w341, w340, w339, w338, w337, w336, w335, w334, w333, w332, w331, w330, w329, w328, w327, w326, w325, w324, w323, w322, w321, w320, w319, w318) -> (w317:refnum<vi>[])
        n158 = call "Strict enable disable.vi"("Disabled"=w316, "Ref in"=w317) -> ()  [unwired: 10 in]
      }
      frame "Hold Update" {
        n159 = call "Hold update .vi"("Enum"=enum16{"Read", "Write"}."Write", "error in (no error)"=w360, "In"=TRUE) -> ("error out"=w359:errorcluster)  [unwired: 7 in, 1 out]
      }
      frame "Update Configuration" {
        n160 = call "File & Folder.vi"("error in (no error)"=w376) -> ("error out"=w371:errorcluster, "File Output"=w375:T4)  [unwired: 9 in]
        n161 = local read "CONFIGURATION FILE"() -> (w373:string)
        n162 = Unbundle By Name(w375) -> ("Configuration path"=w374:path)
        n163 = Build Path(base path=w374, name or relative path=w373) -> (appended path=w372:path)
        n164 = Open/Create/Replace File(file path (use dialog)=w372, error in=w371, prompt="Select file to load", operation (0:open)=T8."open") -> (refnum out=w379:refnum<file>, error out=w370:errorcluster)  [unwired: 2 in, 1 out]
        n165 = Read from Binary File(5:T7 {"AO config"=[], "AI config"=[], "DI config"=[], "DO config"=[], "TC config"=[], "ACC config"=[], "SG config"=[], "Strain Gauge Settings"={"poisson ratio"=0.0, "nominal gage resistance"=120.0, "gage factor"=2.0}, "Bridge Settings"={"voltage excitation value"=3.0, "voltage excitation source"=10200, "initial bridge voltage"=0.0, "lead wire resistance"=1.7, "strain configuration"=10271}, "Sample Rate"={"AI Sample Rate"=[], "AO Sample Rate"=[], "DI Sample Rate"=[], "TC Sample Rate"=[], "DO Sample Rate"=[], "SG Sample Rate"=[], "ACC Sample Rate"=[]}} ("Data"), 8:w370, 11:w379) -> (0:w369:errorcluster, 2:w363:T7, 3:w380:refnum<file>)  [unwired: 3 in, 1 out]
        n166 = Close File(refnum=w380, error in=w369) -> (error out=w367:errorcluster)  [unwired: 1 out]
        n167 = call "Configuration Data.vi"("Enum"=enum16{"Read", "Write"}."Write", "data"=w363) -> ()  [unwired: 8 in, 2 out]
        n168 = call "NS Write.vi"("error in"=w367, "Data"=w363, "Message"=w365) -> ("error out"=w366:errorcluster)  [unwired: 8 in]
      }
      frame "Write DO" {
        n169 = Build Array("F_EPV_131", "F_EPV_132", "F_EPV_136", "F_EPV_21", "F_EPV_41", "N_EPV_68", "N_EPV_ 69", "F_EPV_ 33", "F_EPV_142", "F_EPV_28", "N_EPV_203", "N_EPV_206", "F_EPV_75", "C_EPV_2", "C_EPV_7", "C_EPV_8", "C_EPV_123", "C_EPV_124", "C_EPV_127", "N_EPV_62a", "N_EPV_62b", "N_EPV_61", "G_EPV_51", "N_EPV_141", "C_EPV_803", "C_EPV_18", "C_EPV_1352", "N_EPV_202", "C_EPV_16") -> (w413:bool[])
        n170 = call "NS Write.vi"("error in"=w416, "Data"=w413, "Message"=w414) -> ("error out"=w415:errorcluster)  [unwired: 8 in]
      }
      frame "Update Valve State" {
        n171 = Unbundle(w417) -> ("F_EPV_131"=w446:refnum<vi>, "F_EPV_132"=w445:refnum<vi>, "F_EPV_136"=w444:refnum<vi>, "F_EPV_21"=w443:refnum<vi>, "F_EPV_41"=w442:refnum<vi>, "N_EPV_68"=w441:refnum<vi>, "N_EPV_ 69"=w440:refnum<vi>, "N_EPV_ 33"=w439:refnum<vi>, "F_EPV_142"=w438:refnum<vi>, "F_EPV_28"=w437:refnum<vi>, "N_EPV_203"=w436:refnum<vi>, "N_EPV_206"=w435:refnum<vi>, "F_EPV_75"=w434:refnum<vi>, "C_EPV_2"=w433:refnum<vi>, "C_EPV_7"=w432:refnum<vi>, "C_EPV_8"=w431:refnum<vi>, "C_EPV_123"=w430:refnum<vi>, "C_EPV_124"=w429:refnum<vi>, "C_EPV_127"=w428:refnum<vi>, "N_EPV_62a"=w427:refnum<vi>, "N_EPV_62b"=w426:refnum<vi>, "N_EPV_61"=w425:refnum<vi>, "G_EPV_51"=w424:refnum<vi>, "N_EPV_141"=w423:refnum<vi>, "C_EPV_803"=w422:refnum<vi>, "C_EPV_18"=w421:refnum<vi>, "C_EPV_1352"=w420:refnum<vi>, "N_EPV_202"=w419:refnum<vi>, "C_EPV_16"=w418:refnum<vi>)
        n172 = Build Array(w446, w445, w444, w443, w442, w441, w440, w439, w438, w437, w436, w435, w434, w433, w432, w431, w430, w429, w428, w427, w426, w425, w424, w423, w422, w421, w420, w419, w418) -> (w447:refnum<vi>[])
        n173 = call "Configuration Data.vi"("Enum"=enum16{"Read", "Write"}."Write") -> ("data 2"=w449:T7)  [unwired: 9 in, 1 out]
        n174 = call "Do State extracter.vi"("input cluster"=w449) -> ("Do State"=w448:bool[])  [unwired: 10 in]
        n175 = for {
          tunnel: w448 -> [w454] mode=indexing
          tunnel: w447 -> [w453] mode=indexing
          n176 = property class="Bool (strict)"(reference=w453, "Value"=w454) -> ()  [unwired: 1 in, 2 out]
        }
      }
      frame "Connect RT" {
        n177 = call "NS Main.vi"("error in (no error)"=w462, "Ip Address"="IP ADDRESS") -> ("error out"=w458:errorcluster, "Connected  ?"=w460:bool)  [unwired: 8 in]
        "TARGET" <- w460
        n178 = case shown="True" w460 {
          tunnel: w459 -> [_ w466]
          tunnel: w458 -> [w463 w465]
          tunnel: [w463 w464] -> w457
          frame False {
          }
          frame True {
            n179 = call "Enqueue Message.vi"("error in (no error)"=w465, "Message"="Start", "Message Queue"=w466) -> ("error out"=w464:errorcluster)  [unwired: 7 in, 1 out]
          }
        }
      }
      frame "Connect Drive ATF" {
      }
      frame "Connect Drive LOX" {
      }
      frame "Update Drive ATF Values" {
        n180 = flat-sequence {
          frame #0 {
          }
          frame #1 {
            n181 = One Button Dialog(message="The ATF Drive set parameters are updated .") -> ()  [unwired: 1 in, 1 out]
          }
        }
      }
      frame "Update Drive LOX Values" {
        n182 = flat-sequence {
          frame #0 {
          }
          frame #1 {
            n183 = One Button Dialog(message="The LOX Drive set parameters are updated .") -> ()  [unwired: 1 in, 1 out]
          }
        }
      }
      frame "Gate Driver Power ATF" {
      }
      frame "ADC Reset ATF" {
      }
      frame "MCU Reset ATF" {
      }
      frame "Motor On ATF" {
        w492 = T3 [enum."Disabled and Grayed Out", enum."Disabled and Grayed Out", enum."Disabled and Grayed Out", enum."Disabled and Grayed Out", enum."Disabled and Grayed Out", enum."Enabled"] items=["Enabled", "Disabled", "Disabled and Grayed Out"] ("Disabled")
        n184 = Unbundle By Name(w500) -> ("Update drive ATF"=w499:refnum<vi>, "Gate driver ATF"=w498:refnum<vi>, "ADC reset ATF"=w497:refnum<vi>, "MCU reset ATF"=w496:refnum<vi>, "Motor On ATF"=w495:refnum<vi>, "Motor off ATF"=w494:refnum<vi>)
        n185 = Build Array(w499, w498, w497, w496, w495, w494) -> (w493:refnum<vi>[])
        n186 = call "enable disable.vi"("Disabled"=w492, "ref in"=w493) -> ()  [unwired: 10 in]
      }
      frame "Motor Off ATF" {
        w505 = T3 [enum."Enabled", enum."Enabled", enum."Enabled", enum."Enabled", enum."Enabled", enum."Disabled and Grayed Out"] items=["Enabled", "Disabled", "Disabled and Grayed Out"] ("Disabled")
        n187 = Unbundle By Name(w504) -> ("Update drive ATF"=w503:refnum<vi>, "Gate driver ATF"=w511:refnum<vi>, "ADC reset ATF"=w510:refnum<vi>, "MCU reset ATF"=w509:refnum<vi>, "Motor On ATF"=w508:refnum<vi>, "Motor off ATF"=w507:refnum<vi>)
        n188 = Build Array(w503, w511, w510, w509, w508, w507) -> (w506:refnum<vi>[])
        n189 = call "enable disable.vi"("Disabled"=w505, "ref in"=w506) -> ()  [unwired: 10 in]
      }
      frame "ADC Reset LOX" {
      }
      frame "MCU Reset LOX" {
      }
      frame "Gate Driver Power LOX" {
      }
      frame "Motor On LOX" {
        w523 = T3 [enum."Disabled and Grayed Out", enum."Disabled and Grayed Out", enum."Disabled and Grayed Out", enum."Disabled and Grayed Out", enum."Disabled and Grayed Out", enum."Enabled"] items=["Enabled", "Disabled", "Disabled and Grayed Out"] ("Disabled")
        n190 = Unbundle By Name(w531) -> ("Update drive lox"=w530:refnum<vi>, "Gate driver- LOX"=w529:refnum<vi>, "Adc reset lox"=w528:refnum<vi>, "MCU Reset -LOX"=w527:refnum<vi>, "Motor On lox"=w526:refnum<vi>, "Motor Off lox"=w525:refnum<vi>)
        n191 = Build Array(w530, w529, w528, w527, w526, w525) -> (w524:refnum<vi>[])
        n192 = call "enable disable.vi"("Disabled"=w523, "ref in"=w524) -> ()  [unwired: 10 in]
      }
      frame "Motor Off LOX" {
        w535 = T3 [enum."Enabled", enum."Enabled", enum."Enabled", enum."Enabled", enum."Enabled", enum."Disabled and Grayed Out"] items=["Enabled", "Disabled", "Disabled and Grayed Out"] ("Disabled")
        n193 = Unbundle By Name(w534) -> ("Update drive lox"=w542:refnum<vi>, "Gate driver- LOX"=w541:refnum<vi>, "Adc reset lox"=w540:refnum<vi>, "MCU Reset -LOX"=w539:refnum<vi>, "Motor On lox"=w538:refnum<vi>, "Motor Off lox"=w537:refnum<vi>)
        n194 = Build Array(w542, w541, w540, w539, w538, w537) -> (w536:refnum<vi>[])
        n195 = call "enable disable.vi"("Disabled"=w535, "ref in"=w536) -> ()  [unwired: 10 in]
      }
      frame "Connect PPSU" {
      }
      frame "DC ON PPSU" {
        w548 = T3 [enum."Disabled and Grayed Out", enum."Disabled and Grayed Out", enum."Disabled and Grayed Out", enum."Disabled and Grayed Out", enum."Enabled"] items=["Enabled", "Disabled", "Disabled and Grayed Out"] ("Disabled")
        n196 = Unbundle By Name(w555) -> ("update ppsu"=w554:refnum<vi>, "Alarm ack"=w553:refnum<vi>, "Ms initialize"=w552:refnum<vi>, "DC on"=w551:refnum<vi>, "DC off"=w550:refnum<vi>)
        n197 = Build Array(w554, w553, w552, w551, w550) -> (w549:refnum<vi>[])
        n198 = call "enable disable.vi"("Disabled"=w548, "ref in"=w549) -> ()  [unwired: 10 in]
      }
      frame "DC OFF PPSU" {
        w559 = T3 [enum."Enabled", enum."Enabled", enum."Enabled", enum."Enabled", enum."Disabled and Grayed Out"] items=["Enabled", "Disabled", "Disabled and Grayed Out"] ("Disabled")
        n199 = Unbundle By Name(w558) -> ("update ppsu"=w565:refnum<vi>, "Alarm ack"=w564:refnum<vi>, "Ms initialize"=w563:refnum<vi>, "DC on"=w562:refnum<vi>, "DC off"=w561:refnum<vi>)
        n200 = Build Array(w565, w564, w563, w562, w561) -> (w560:refnum<vi>[])
        n201 = call "enable disable.vi"("Disabled"=w559, "ref in"=w560) -> ()  [unwired: 10 in]
      }
      frame "Update PPSU Values" {
        n202 = flat-sequence {
          frame #0 {
          }
          frame #1 {
            n203 = One Button Dialog(message="The PPSU set parameters are updated.") -> ()  [unwired: 1 in, 1 out]
          }
        }
      }
      frame "Alarm Ack PPSU" {
      }
      frame "MS Initialize PPSU" {
      }
      frame "RT Exit" {
      }
      frame "Exit" {
        n204 = Unbundle By Name(w590) -> ("Data"=w589:refnum<notifier>)
        n205 = call "Enqueue Message.vi"("error in (no error)"=w585, "Message"="Exit", "Message Queue"=w583) -> ("error out"=w584:errorcluster)  [unwired: 7 in, 1 out]
        n206 = Release Queue(queue=w593, error in (no error)=w584) -> (error out=w588:errorcluster)  [unwired: 1 in, 2 out]
        n207 = Release Queue(queue=w583, error in (no error)=w588) -> (error out=w587:errorcluster)  [unwired: 1 in, 2 out]
        n208 = call "Fire User Event - Stop.vi"("error in (no error)"=w587, "User Event - Stop"=w594) -> ("error out"=w586:errorcluster)  [unwired: 9 in]
        n209 = Release Notifier(notifier=w589, error in (no error)=w586) -> (error out=w592:errorcluster)  [unwired: 1 in, 2 out]
        n210 = global write "Phase III Globals.vi" "Exit"(TRUE ("Exit")) -> ()
      }
      frame "Phase Code Name" {
        n211 = call "Phase code name.vi"("Enum"=enum16{"Read", "Write"}."Write", "error in"=w599, "Phase code W"="Datalog phase code") -> ("error out"=w598:errorcluster)  [unwired: 7 in, 1 out]
      }
      frame "Select Configuration" {
        n212 = call "Configuration File Name.vi"("Enum"=enum16{"Read", "Write"}."Write", "error in"=w605, "Phase code W"="CONFIGURATION FILE") -> ("error out"=w603:errorcluster)  [unwired: 7 in, 1 out]
      }
      frame "Daq Setting" {
        n213 = call "File & Folder.vi"("error in (no error)"=w624) -> ("error out"=w623:errorcluster, "File Output"=w622:T4)  [unwired: 9 in]
        n214 = Unbundle By Name(w622) -> ("Configuration path"=w615:path, "Sub vi's"=w621:path)
        n215 = Build Path(base path=w621, name or relative path=path "Hardware Config.vi") -> (appended path=w619:path)
        n216 = call "Call by reference.vi"("error in"=w623, "vi path"=w619) -> ("error out"=w616:errorcluster)  [unwired: 9 in]
        n217 = List Folder(path=w615, error in=w616) -> (filenames=w614:string[], error out=w609:errorcluster)  [unwired: 2 in, 2 out]
        n218 = control-ref of="CONFIGURATION FILE"() -> (w617:refnum<vi>)
        n219 = call "Configuration File Name.vi"("Enum"=enum16{"Read", "Write"}."Read", "error in"=w609) -> ("error out"=w608:errorcluster, "Phase codeR"=w610:string)  [unwired: 8 in]
        n220 = property class="CmbBox"(reference=w617, error in=w608, "Strings[]"=w614, "Value"=w610) -> (error out=w613:errorcluster)  [unwired: 1 out]
      }
      frame "Abort" {
      }
      frame "Add User" {
        n221 = call "Add_User P3.vi"("error in (no error)"=w629) -> ("error out"=w628:errorcluster)  [unwired: 10 in]
      }
    }
    n222 = call "UI Error Handler - Message Handler.vi"("error in (no error)"=w135, "Message Queue"=w136) -> ()  [unwired: 9 in, 1 out]
    n223 = call <vilib>:"Clear Errors.vi"("error in (no error)"=w135) -> ("error out"=w146:errorcluster)  [unwired: 5 in, 1 out]
  }
  n224 = call "NS Reader.vi"("error in"=w9, "notifier in"=w10, "Message Queues in"=w11) -> ("error out"=w8:errorcluster)  [unwired: 7 in, 1 out]
  n225 = while {
    tunnel: w15 -> [w644]
    stop <- w640 stop-if-true
    # "Healths"
    # "Drive LOX"
    # "PPSU"
    # "DI Data"
    # "ATF Drive"
    # "Monitoring Loop"
    n226 = Get Date/Time In Seconds() -> (seconds since 1Jan1904=→"Time Stamp":timestamp)
    n227 = Wait on Notification(notifier=w644, timeout in ms (-1)=100) -> (error out=w641:errorcluster)  [unwired: 2 in, 3 out]
    n228 = Or(x=w641, y="EXIT") -> (x .or. y?=w640:bool)
    n229 = call "Log Health.vi"("Enum"=enum16{"Read", "Write"}."Read") -> ("Log health R"=→"LOG":bool)  [unwired: 9 in, 1 out]
    n230 = call "DI Search Channel.vi"() -> ("Array 2"=w636:bool[])  [unwired: 11 in]
    n231 = Index Array(array=w636) -> (element=→"F_EPV_131 HSS":bool)  [unwired: 1 in]
    n232 = Wait Until Next ms Multiple(millisecond multiple=u32 100) -> ()  [unwired: 1 out]
    "User 2" <- "-------" ("User 2")
    "User 3" <- "--------" ("User 3")
  }
  n233 = call "Queue Data log module.vi"("error in"=w9) -> ("error out"=w13:errorcluster)  [unwired: 10 in]
  n234 = while {
    tunnel: w26 -> [w653]
    tunnel: [w652] -> w25
    tunnel: w19 -> [w651]
    shift-right: [w649] -> w18
    shift-left: w9 -> [w650]
    stop <- w645 stop-if-true
    # "Event Loop"
    n235 = event shown="[11] \"Log In Tool\": Value Change" {
      selector: w653 -> [_ _ _ _ _ _ _ _ _ _ _ _ _ _ _ _ _ _ _ _ _ _ _ _ _ _ _ _ _ _ _ _ _ _ _ _ _]
      dyn-events: [_ _ _ _ _ _ _ _ _ _ _ _ _ _ _ _ _ _ _ _ _ _ _ _ _ _ _ _ _ _ _ _ _ _ _ _ _] -> w652
      timeout: _ -> [_ _ _ _ _ _ _ _ _ _ _ _ _ _ _ _ _ _ _ _ _ _ _ _ _ _ _ _ _ _ _ _ _ _ _ _ _]
      tunnel: [_ _ _ _ TRUE _ _ _ _ _ _ _ _ _ _ _ _ _ _ _ _ _ _ _ _ _ _ _ _ _ _ _ _ _ _ _ _] -> w646
      tunnel: w651 -> [w663 w666 w674 w684 w690 w699 w703 w710 w713 w720 w726 w731 w734 w741 w743 w748 w756 w758 w763 w768 w774 w778 w783 w788 w792 w799 w802 w808 w814 w820 w824 w829 w834 w839 w844 w849 w856]
      tunnel: w650 -> [w662 w668 w675 w686 w692 w698 w705 w707 w715 w719 w723 w730 w736 w740 w746 w751 w754 w760 w766 w770 w776 w780 w786 w791 w795 w801 w805 w810 w816 w819 w826 w831 w836 w841 w846 w851 w855]
      tunnel: [w662 w667 w681 w685 w691 w697 w704 w708 w714 w718 w722 w729 w735 w739 w745 w750 w753 w759 w765 w769 w775 w779 w785 w790 w794 w800 w804 w809 w815 w818 w825 w830 w835 w840 w845 w850 w854] -> w648
      tunnel: [w663 w664 w679 w682 w688 w696 w702 w709 w712 w717 w721 w728 w733 w738 w744 w749 w755 w757 w764 w767 w773 w777 w784 w787 w793 w798 w803 w807 w813 w817 w823 w828 w833 w838 w843 w848 w853] -> w647
      event Timeout {
        n236 = event-data() -> ()  [unwired: 1 in, 3 out]
      }
      event "F_EPV_131", "F_EPV_136", "F_EPV_132", "F_EPV_21", "F_EPV_41", "N_EPV_68", "N_EPV_ 69", "F_EPV_ 33", "F_EPV_142", "F_EPV_28", "N_EPV_203", "N_EPV_206", "F_EPV_75", "C_EPV_2", "C_EPV_7", "C_EPV_8", "C_EPV_123", "C_EPV_127", "N_EPV_62a", "N_EPV_62b", "N_EPV_61", "G_EPV_51", "N_EPV_141", "C_EPV_803", "C_EPV_18", "C_EPV_1352", "N_EPV_202", "C_EPV_16", "C_EPV_124": Value Change {
        n237 = event-data() -> ()  [unwired: 1 in, 3 out]
        n238 = call "Enqueue Message.vi"("error in (no error)"=w668, "Message"="Write DO", "Message Queue"=w666) -> ("error out"=w667:errorcluster, "dup Message Queue"=w664:refnum<queue>)  [unwired: 7 in]
      }
      event "START DAQ": Value Change {
        n239 = event-data() -> ()  [unwired: 1 in, 1 out]
        n240 = call "Enqueue Message.vi"("error in (no error)"=w675, "Message"="Update Configuration", "Message Queue"=w674) -> ("error out"=w672:errorcluster, "dup Message Queue"=w671:refnum<queue>)  [unwired: 7 in]
        n241 = call "Enqueue Message.vi"("error in (no error)"=w672, "Message"="Update Valve Statete Configuration", "Message Queue"=w671) -> ("error out"=w669:errorcluster, "dup Message Queue"=w670:refnum<queue>)  [unwired: 7 in]
        n242 = To Variant(anything=bool[] [TRUE, FALSE]) -> (Variant=w677:variant)
        n243 = call "Enqueue Message.vi"("error in (no error)"=w669, "Message Data"=w677, "Message"="Start Daq", "Message Queue"=w670) -> ("error out"=w681:errorcluster, "dup Message Queue"=w679:refnum<queue>)  [unwired: 6 in]
      }
      event "START LOG": Value Change {
        n244 = event-data() -> ()  [unwired: 1 in, 3 out]
        n245 = call "Enqueue Message.vi"("error in (no error)"=w686, "Message"="Start Datalog", "Message Queue"=w684) -> ("error out"=w685:errorcluster, "dup Message Queue"=w682:refnum<queue>)  [unwired: 7 in]
      }
      event "EXIT": Value Change {
        n246 = event-data() -> ()  [unwired: 1 in, 1 out]
        n247 = call "Enqueue Message.vi"("Priority Message? (F)"=TRUE, "error in (no error)"=w692, "Message"="Exit", "Message Queue"=w690) -> ("error out"=w691:errorcluster, "dup Message Queue"=w688:refnum<queue>)  [unwired: 6 in]
      }
      event "STOP DAQ": Value Change {
        n248 = event-data() -> ()  [unwired: 1 in, 1 out]
        n249 = To Variant(anything=bool[] [FALSE, TRUE]) -> (Variant=w694:variant)
        n250 = call "Enqueue Message.vi"("error in (no error)"=w698, "Message Data"=w694, "Message"="Stop Daq", "Message Queue"=w699) -> ("error out"=w697:errorcluster, "dup Message Queue"=w696:refnum<queue>)  [unwired: 6 in]
      }
      event "Connect RT": Value Change {
        n251 = event-data() -> ()  [unwired: 1 in, 2 out]
        n252 = call "Enqueue Message.vi"("error in (no error)"=w705, "Message"="Connect RT", "Message Queue"=w703) -> ("error out"=w704:errorcluster, "dup Message Queue"=w702:refnum<queue>)  [unwired: 7 in]
      }
      event "Connect ppsu": Value Change {
        n253 = event-data() -> ()  [unwired: 1 in, 3 out]
        n254 = call "Enqueue Message.vi"("error in (no error)"=w707, "Message"="Connect PPSU", "Message Queue"=w710) -> ("error out"=w708:errorcluster, "dup Message Queue"=w709:refnum<queue>)  [unwired: 7 in]
      }
      event "DAQ SETTING": Value Change {
        n255 = event-data() -> ()  [unwired: 1 in, 1 out]
        n256 = call "Enqueue Message.vi"("error in (no error)"=w715, "Message"="Daq Setting", "Message Queue"=w713) -> ("error out"=w714:errorcluster, "dup Message Queue"=w712:refnum<queue>)  [unwired: 7 in]
      }
      event "HOLD UPDATE": Value Change {
        n257 = event-data() -> ()  [unwired: 1 in, 1 out]
        n258 = call "Enqueue Message.vi"("error in (no error)"=w719, "Message"="Hold Update", "Message Queue"=w720) -> ("error out"=w718:errorcluster, "dup Message Queue"=w717:refnum<queue>)  [unwired: 7 in]
      }
      event "IP ADDRESS": Value Change {
        n259 = event-data() -> ("NewVal"=w725:string)  [unwired: 1 in]
        n260 = call "Enqueue Message.vi"("error in (no error)"=w723, "Message Data"=w725, "Message"="Ip Config", "Message Queue"=w726) -> ("error out"=w722:errorcluster, "dup Message Queue"=w721:refnum<queue>)  [unwired: 6 in]
      }
      event "Log In Tool": Value Change {
        n261 = event-data() -> ()  [unwired: 1 in, 5 out]
        n262 = call "Enqueue Message.vi"("error in (no error)"=w730, "Message"="Add User", "Message Queue"=w731) -> ("error out"=w729:errorcluster, "dup Message Queue"=w728:refnum<queue>)  [unwired: 7 in]
      }
      event "CONFIGURATION FILE": Value Change {
        n263 = event-data() -> ()  [unwired: 1 in, 1 out]
        n264 = call "Enqueue Message.vi"("error in (no error)"=w736, "Message"="Select Configuration", "Message Queue"=w734) -> ("error out"=w735:errorcluster, "dup Message Queue"=w733:refnum<queue>)  [unwired: 7 in]
      }
      event "ABORT": Value Change {
        n265 = event-data() -> ()  [unwired: 1 in, 1 out]
        n266 = call "Enqueue Message.vi"("error in (no error)"=w740, "Message"="Abort", "Message Queue"=w741) -> ("error out"=w739:errorcluster, "dup Message Queue"=w738:refnum<queue>)  [unwired: 7 in]
      }
      event "Datalog phase code": Value Change {
        n267 = event-data() -> ()  [unwired: 1 in, 6 out]
        n268 = call "Enqueue Message.vi"("error in (no error)"=w746, "Message"="Phase Code Name", "Message Queue"=w743) -> ("error out"=w745:errorcluster, "dup Message Queue"=w744:refnum<queue>)  [unwired: 7 in]
      }
      event "Connect Drive ATF": Value Change {
        n269 = event-data() -> ()  [unwired: 1 in, 6 out]
        n270 = call "Enqueue Message.vi"("error in (no error)"=w751, "Message"="Connect Drive ATF", "Message Queue"=w748) -> ("error out"=w750:errorcluster, "dup Message Queue"=w749:refnum<queue>)  [unwired: 7 in]
      }
      event "Connect Drive Lox": Value Change {
        n271 = event-data() -> ()  [unwired: 1 in, 1 out]
        n272 = call "Enqueue Message.vi"("error in (no error)"=w754, "Message"="Connect Drive LOX", "Message Queue"=w756) -> ("error out"=w753:errorcluster, "dup Message Queue"=w755:refnum<queue>)  [unwired: 7 in]
      }
      event "Alarm ack": Value Change {
        n273 = event-data() -> ()  [unwired: 1 in, 4 out]
        n274 = call "Enqueue Message.vi"("error in (no error)"=w760, "Message"="Alarm Ack PPSU", "Message Queue"=w758) -> ("error out"=w759:errorcluster, "dup Message Queue"=w757:refnum<queue>)  [unwired: 7 in]
      }
      event "Ms initialize": Value Change {
        n275 = event-data() -> ()  [unwired: 1 in, 4 out]
        n276 = call "Enqueue Message.vi"("error in (no error)"=w766, "Message"="MS Initialize PPSU", "Message Queue"=w763) -> ("error out"=w765:errorcluster, "dup Message Queue"=w764:refnum<queue>)  [unwired: 7 in]
      }
      event "update ppsu": Value Change {
        n277 = event-data() -> ()  [unwired: 1 in, 4 out]
        n278 = call "Enqueue Message.vi"("error in (no error)"=w770, "Message"="Update PPSU Values", "Message Queue"=w768) -> ("error out"=w769:errorcluster, "dup Message Queue"=w767:refnum<queue>)  [unwired: 7 in]
      }
      event "Update drive ATF": Value Change {
        n279 = event-data() -> ()  [unwired: 1 in, 4 out]
        n280 = call "Enqueue Message.vi"("error in (no error)"=w776, "Message"="Update Drive ATF Values", "Message Queue"=w774) -> ("error out"=w775:errorcluster, "dup Message Queue"=w773:refnum<queue>)  [unwired: 7 in]
      }
      event "STOP LOG": Value Change {
        n281 = event-data() -> ()  [unwired: 1 in, 4 out]
        n282 = call "Enqueue Message.vi"("error in (no error)"=w780, "Message"="Stop Datalog", "Message Queue"=w778) -> ("error out"=w779:errorcluster, "dup Message Queue"=w777:refnum<queue>)  [unwired: 7 in]
      }
      event "Update drive lox": Value Change {
        n283 = event-data() -> ()  [unwired: 1 in, 4 out]
        n284 = call "Enqueue Message.vi"("error in (no error)"=w786, "Message"="Update Drive LOX Values", "Message Queue"=w783) -> ("error out"=w785:errorcluster, "dup Message Queue"=w784:refnum<queue>)  [unwired: 7 in]
      }
      event "Motor On lox": Value Change {
        n285 = event-data() -> ()  [unwired: 1 in, 4 out]
        n286 = call "Enqueue Message.vi"("error in (no error)"=w791, "Message"="Motor On LOX", "Message Queue"=w788) -> ("error out"=w790:errorcluster, "dup Message Queue"=w787:refnum<queue>)  [unwired: 7 in]
      }
      event "Motor Off lox": Value Change {
        n287 = event-data() -> ()  [unwired: 1 in, 4 out]
        n288 = call "Enqueue Message.vi"("error in (no error)"=w795, "Message"="Motor Off LOX", "Message Queue"=w792) -> ("error out"=w794:errorcluster, "dup Message Queue"=w793:refnum<queue>)  [unwired: 7 in]
      }
      event "DC on": Value Change {
        n289 = event-data() -> ()  [unwired: 1 in, 4 out]
        n290 = call "Enqueue Message.vi"("error in (no error)"=w801, "Message"="DC ON PPSU", "Message Queue"=w799) -> ("error out"=w800:errorcluster, "dup Message Queue"=w798:refnum<queue>)  [unwired: 7 in]
      }
      event "DC off": Value Change {
        n291 = event-data() -> ()  [unwired: 1 in, 4 out]
        n292 = call "Enqueue Message.vi"("error in (no error)"=w805, "Message"="DC OFF PPSU", "Message Queue"=w802) -> ("error out"=w804:errorcluster, "dup Message Queue"=w803:refnum<queue>)  [unwired: 7 in]
      }
      event "Gate driver- LOX": Value Change {
        n293 = event-data() -> ()  [unwired: 1 in, 4 out]
        n294 = call "Enqueue Message.vi"("error in (no error)"=w810, "Message"="Gate Driver Power LOX", "Message Queue"=w808) -> ("error out"=w809:errorcluster, "dup Message Queue"=w807:refnum<queue>)  [unwired: 7 in]
      }
      event "MCU Reset -LOX": Value Change {
        n295 = event-data() -> ()  [unwired: 1 in, 4 out]
        n296 = call "Enqueue Message.vi"("error in (no error)"=w816, "Message"="MCU Reset LOX", "Message Queue"=w814) -> ("error out"=w815:errorcluster, "dup Message Queue"=w813:refnum<queue>)  [unwired: 7 in]
      }
      event "Adc reset lox": Value Change {
        n297 = event-data() -> ()  [unwired: 1 in, 4 out]
        n298 = call "Enqueue Message.vi"("error in (no error)"=w819, "Message"="ADC Reset LOX", "Message Queue"=w820) -> ("error out"=w818:errorcluster, "dup Message Queue"=w817:refnum<queue>)  [unwired: 7 in]
      }
      event "Motor On ATF": Value Change {
        n299 = event-data() -> ()  [unwired: 1 in, 4 out]
        n300 = call "Enqueue Message.vi"("error in (no error)"=w826, "Message"="Motor On ATF", "Message Queue"=w824) -> ("error out"=w825:errorcluster, "dup Message Queue"=w823:refnum<queue>)  [unwired: 7 in]
      }
      event "Motor off ATF": Value Change {
        n301 = event-data() -> ()  [unwired: 1 in, 4 out]
        n302 = call "Enqueue Message.vi"("error in (no error)"=w831, "Message"="Motor Off ATF", "Message Queue"=w829) -> ("error out"=w830:errorcluster, "dup Message Queue"=w828:refnum<queue>)  [unwired: 7 in]
      }
      event "Gate driver ATF": Value Change {
        n303 = event-data() -> ()  [unwired: 1 in, 4 out]
        n304 = call "Enqueue Message.vi"("error in (no error)"=w836, "Message"="Gate Driver Power ATF", "Message Queue"=w834) -> ("error out"=w835:errorcluster, "dup Message Queue"=w833:refnum<queue>)  [unwired: 7 in]
      }
      event "MCU reset ATF": Value Change {
        n305 = event-data() -> ()  [unwired: 1 in, 4 out]
        n306 = call "Enqueue Message.vi"("error in (no error)"=w841, "Message"="MCU Reset ATF", "Message Queue"=w839) -> ("error out"=w840:errorcluster, "dup Message Queue"=w838:refnum<queue>)  [unwired: 7 in]
      }
      event "ADC reset ATF": Value Change {
        n307 = event-data() -> ()  [unwired: 1 in, 4 out]
        n308 = call "Enqueue Message.vi"("error in (no error)"=w846, "Message"="ADC Reset ATF", "Message Queue"=w844) -> ("error out"=w845:errorcluster, "dup Message Queue"=w843:refnum<queue>)  [unwired: 7 in]
      }
      event "Exit RT": Value Change {
        n309 = event-data() -> ()  [unwired: 1 in, 4 out]
        n310 = call "Enqueue Message.vi"("error in (no error)"=w851, "Message"="RT Exit", "Message Queue"=w849) -> ("error out"=w850:errorcluster, "dup Message Queue"=w848:refnum<queue>)  [unwired: 7 in]
      }
      event "Configure IP": Value Change {
        n311 = event-data() -> ()  [unwired: 1 in, 4 out]
        n312 = call "Enqueue Message.vi"("error in (no error)"=w855, "Message"="Ip Config", "Message Queue"=w856) -> ("error out"=w854:errorcluster, "dup Message Queue"=w853:refnum<queue>)  [unwired: 7 in]
      }
    }
    n313 = case shown="Error .." w648 {
      selector: w648 -> [w657 _]
      tunnel: [w657 _] -> w649
      tunnel: w647 -> [_ w660]
      tunnel: w646 -> [w656 _]
      tunnel: [w654 TRUE] -> w645
      frame No Error {
        n314 = global read "Phase III Globals.vi" "Exit"() -> (w655:bool)
        n315 = Or(x=w655, y=w656) -> (x .or. y?=w654:bool)
      }
      frame Error {
        n316 = call "Enqueue Message.vi"("Priority Message? (F)"=TRUE, "Message"="Exit", "Message Queue"=w660) -> ()  [unwired: 7 in, 2 out]
      }
    }
  }
  n317 = call "Destroy User Event - Stop.vi"("error in (no error)"=w14, "User Event - Stop"=w21) -> ("error out"=w22:errorcluster)  [unwired: 9 in]
  n318 = Unregister For Events(event registration refnum=w25, error in=w18) -> (error out=w24:errorcluster)
  n319 = Merge Errors(w13, w24, w22, w8) -> (w12:errorcluster)
  n320 = call <vilib>:"Simple Error Handler.vi"("error in (no error)"=w12) -> ()  [unwired: 4 in, 5 out]
